vi "SpectrometerSpinCoater_v03_HardwareTrigger.vi"() -> ()   [LabVIEW 2018]
uses:
  <instrlib>/Classes/CCD/Abstract_CCD/Abstract_CCD.lvclass
  TypDef/DeviceQueue_TypeDef.ctl
  TypDef/DeviceQueue_Action.ctl
  TypDef/DataQueue_TypeDef.ctl
  TypDef/DataQueue_Action.ctl
  <vilib>/Utility/error.llb/DialogType.ctl
  <instrlib>/Classes/CCD/Avantes/Avantes.lvclass
  C:/Program Files/National Instruments/LabVIEW 2018/instr.lib/Classes/CCD/Abstract_CCD/Abstract_CCD.lvclass
  <vilib>/Instr/_visa.llb/VISA Configure Serial Port (Instr).vi
panel:
  out "Time.spin":refnum<file>
  out "Meas.spin":refnum<file>
  out "Arduino":bool
  out "NKT":bool
  out "Spectromter":bool
  in  "Abort Button":bool
  in  "Stop Button":bool
  in  "Tab Control":enum32{"Measure", "Settings"}(tab)=enum."Settings"
  out "Action":string
  in  "Preview":bool
  out "XY Graph":T1(graph)
  in  "Frames for Dark/Ref":dbl=1.0
  in  "StartSpin_Button":bool
  out "Overall Time":dbl
  in  "Seconds after Spin Stop":dbl[unit]=0.5
  in  "Program Spin Coater\nSpeed (rpm)          Time (s)":dbl[][](array[numeric])
  in  "Record RefSpec":bool
  in  "Record_Darkspec":bool
  in  "Comments":string="Just for testing"
  in  "File Name":string="Temp"
  in  "Save Path":path=path "C:/Users/Timo/Desktop/SpinCoater/Measurement"
  in  "Seconds to Spin Start":dbl[unit]=1.0
  in  "Calculate Frames":bool=TRUE
  in  "Frames":i32
  out "Frame Rate":dbl[unit]
  in  "Integration Time":dbl[unit]=3e-05
  in  "StartMeasurement_Button":bool
  in  "Speed":dbl
  in  "Milliseconds":dbl
  in  "Debug":bool
  in  "Port Arduino":refnum<visa-resource-name>="COM6"
  out "Error Arduino":bool caption="Error"
  in  "Init_Arduino":bool=TRUE caption="Init"
  out "Caption_Settings_Arduino":string="Arduino"
  out "Caption_Settings_NKT":string="NKT Laser"
  out "Error_Spectromter":bool caption="Error"
  in  "Init_Spectrometer":bool=TRUE caption="Init"
  out "Caption_Settings_Spectrometer":string="Spectromter"
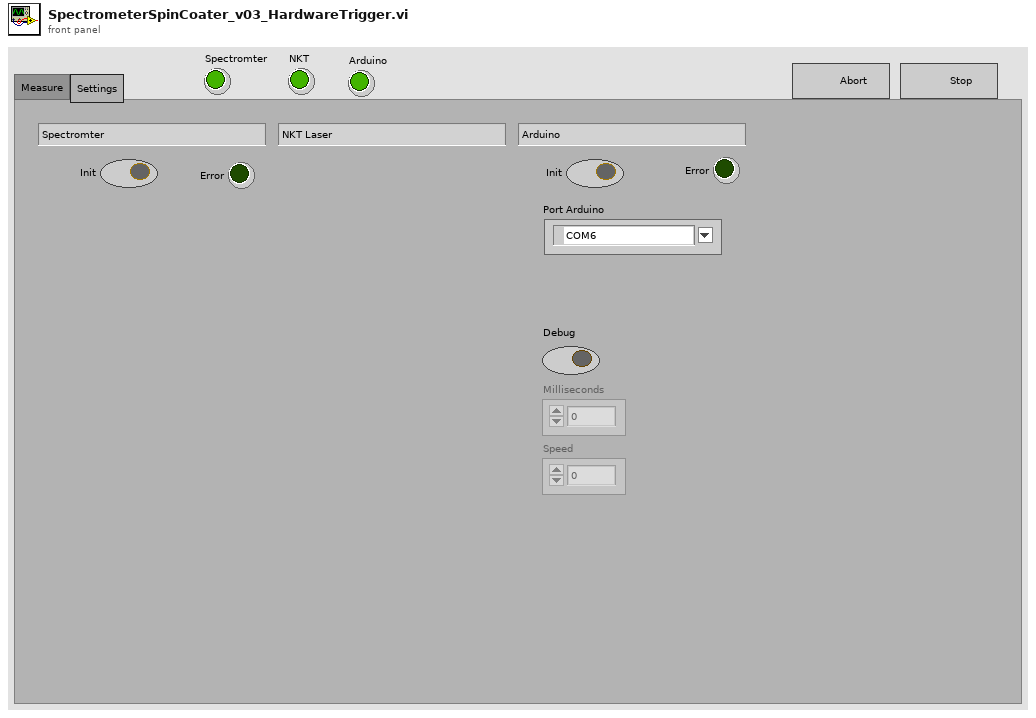
[diagram p1: front panel]
types:
  T1 = cluster{"Wavlength":dbl[unit][], "Image":dbl[]}[]
  T2 = cluster{"Dark":cluster{"Image":dbl[][][], "Frame Size":cluster{"F":i32, "Y":i32, "X":i32}}[], "Ref":cluster{"Image":dbl[][][], "Frame Size":cluster{"F":i32, "Y":i32, "X":i32}}[], "Wavlength":dbl[unit][], "spec":dbl[][]}
  T3 = cluster{"Port Arduino":refnum<visa-resource-name>, "Abstract_CCD.lvclass":refnum<class "Abstract_CCD.lvclass">}
  T4 = typedef "DataQueue_TypeDef.ctl" = cluster{"QueueAction":T5, "Data":cluster{"Image":dbl[][][], "Frame Size":cluster{"F":i32, "Y":i32, "X":i32}}[], "Data_Raw":cluster{"Image":dbl[][][], "Frame Size":cluster{"F":i32, "Y":i32, "X":i32}}[], "Data_Dark":cluster{"Image":dbl[][][], "Frame Size":cluster{"F":i32, "Y":i32, "X":i32}}[], "Data_Ref":cluster{"Image":dbl[][][], "Frame Size":cluster{"F":i32, "Y":i32, "X":i32}}[], "Device Information":string[], "Numeric Control":dbl, "Boolean":bool, "Wavelength":dbl[unit][], "Time":dbl[], "Time Stamp":timestamp, "Numeric Control 2":dbl}
  T5 = typedef "DataQueue_Action.ctl" = enum16{"TimeOut", "Close_Program", "Stop_Measurement", "Measure_InSituSpinCoating", "Save_Data", "Set_Ref", "Set_Dark", "Set_Wavelength", "Spectrometer_Measure", "Transfer_Settings"}
  T6 = typedef "DeviceQueue_TypeDef.ctl" = cluster{"QueueAction":T7, "Numeric 1":dbl, "Numeric 2":dbl, "Boolean 1":bool, "Boolean 2":bool, "Spin Program":dbl[][]}
  T7 = typedef "DeviceQueue_Action.ctl" = enum16{"TimeOut", "Close_Program", "Abort", "Spectrometer_Init", "Spectrometer_Close", "Spectrometer_StartMeasurement", "Spectrometer_StopMeasurement", "Spectrometer_GetData", "Spectrometer_Measure", "Spectrometer_Preview", "Spectrometer_Abort", "Spectrometer_SetIntegrationTime", "Spectrometer_SetFrames", "Spectrometer_SetDarkspec", "Spectrometer_SetReference", "Spectrometer_SetTriggerMode", "Spectrometer_DeviceInformation", "Laser_Init", "Laser_Close", "Arduino_Init", "Arduino_Close", "Arduino_LoadProgram", "Arduino_StartProgram", "Arduino_SetSpeed", "Arduino_SetMillis", "Arduino_StopSpin", "Measure_InSitu", "Measure_Stop"}
  T8 = enum16{"open", "replace", "create", "open or create", "replace or create", "replace or create with confirmation"}
  T9 = cluster{"Image":dbl[][][], "Frame Size":cluster{"F":i32, "Y":i32, "X":i32}}[]
  T10 = cluster{"Image":dbl[][][], "Frame Size":cluster{"F":i32, "Y":i32, "X":i32}}
  T11 = cluster{"Image":dbl[], "Image":dbl[], dbl[], "Numeric Control":dbl, "Numeric Control 2":dbl}
  T12 = typedef "DialogType.ctl" = u16
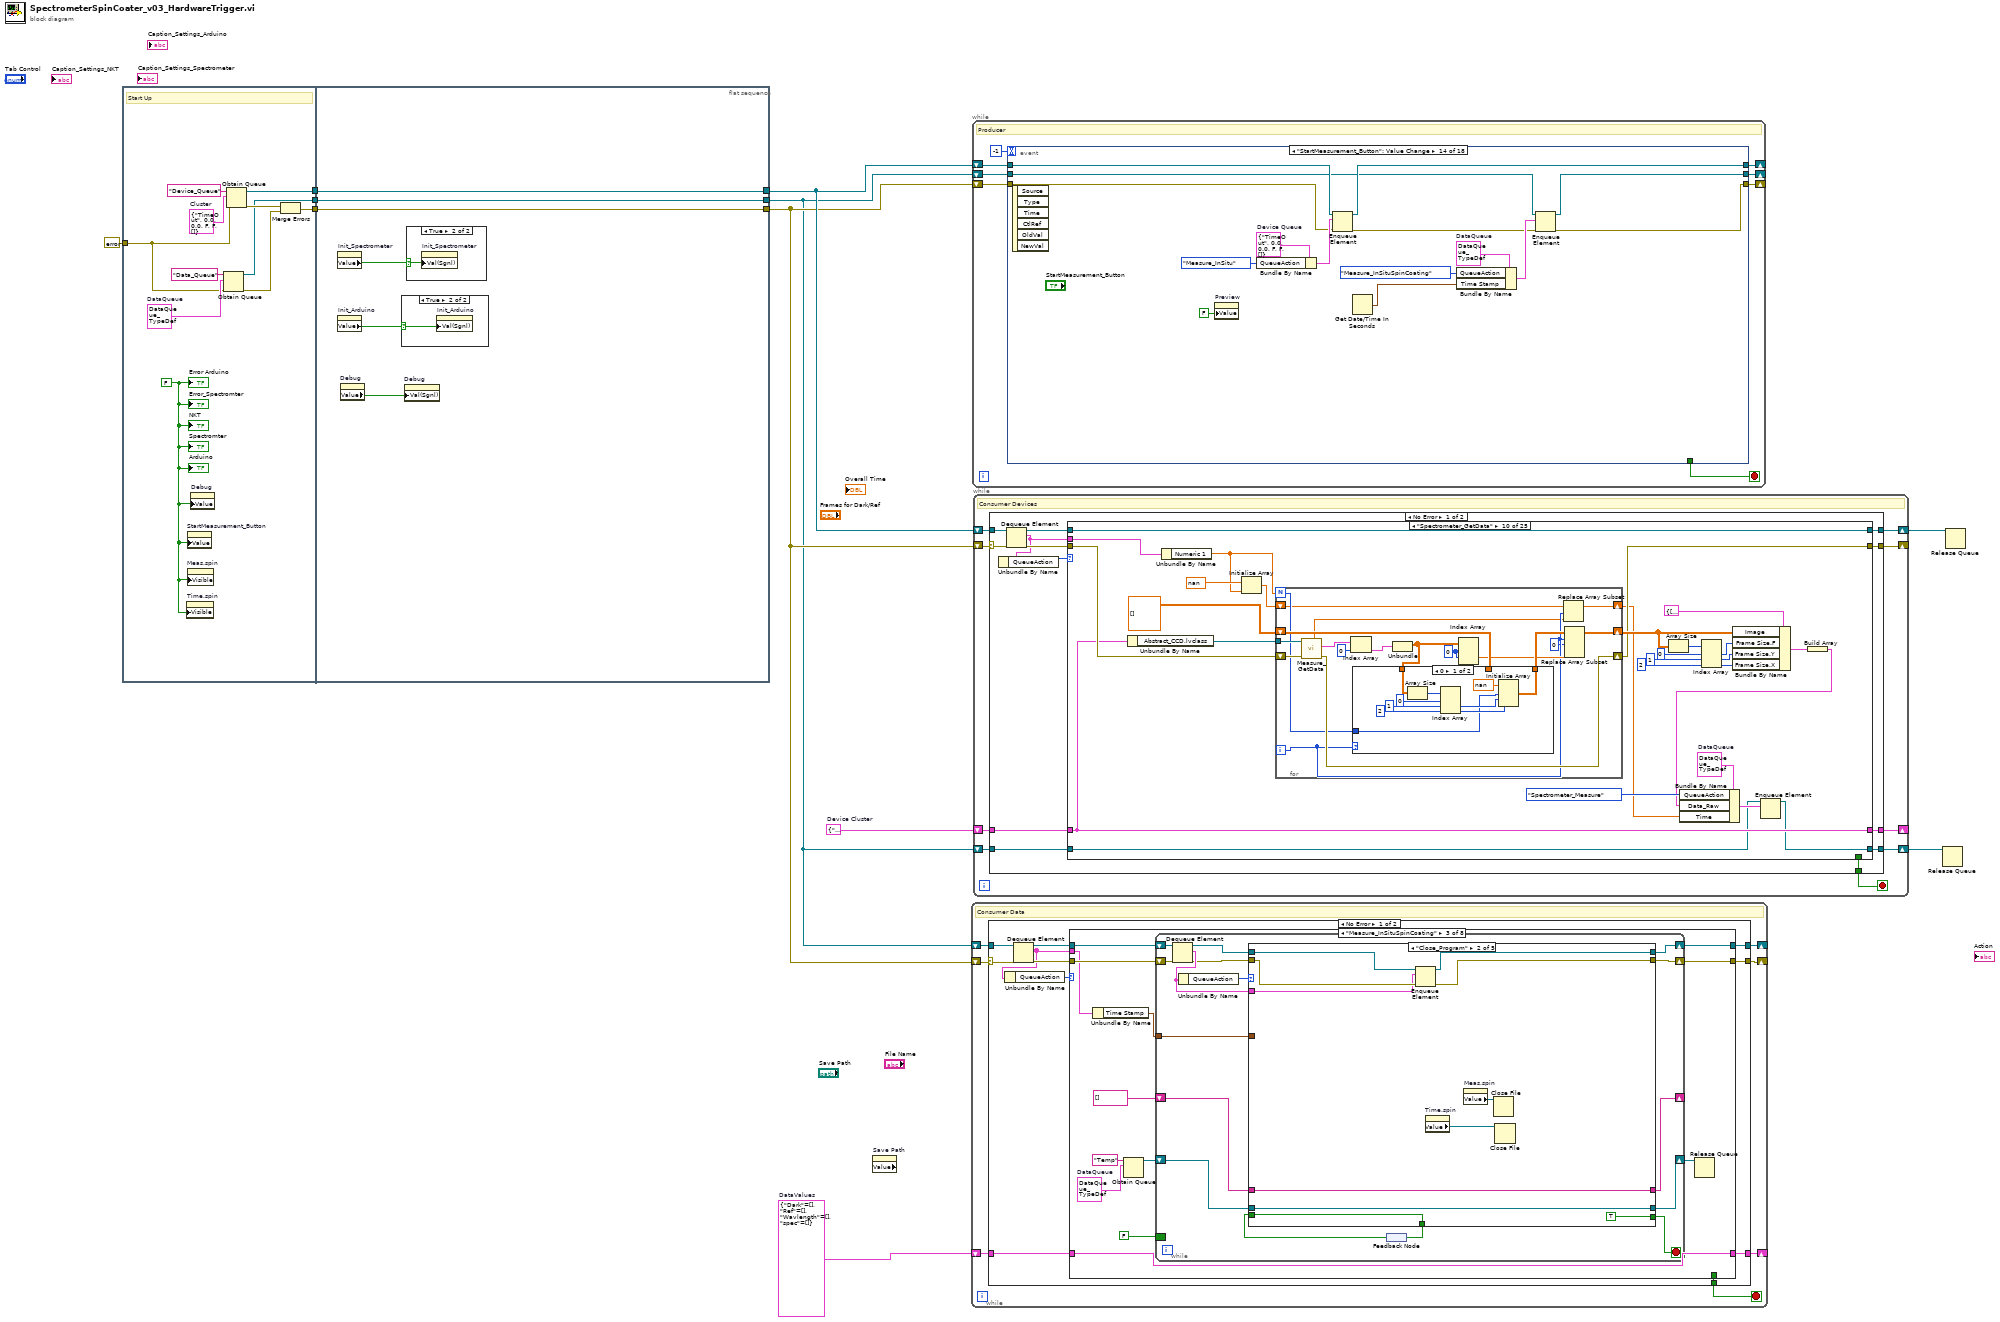
[diagram p0: block diagram]
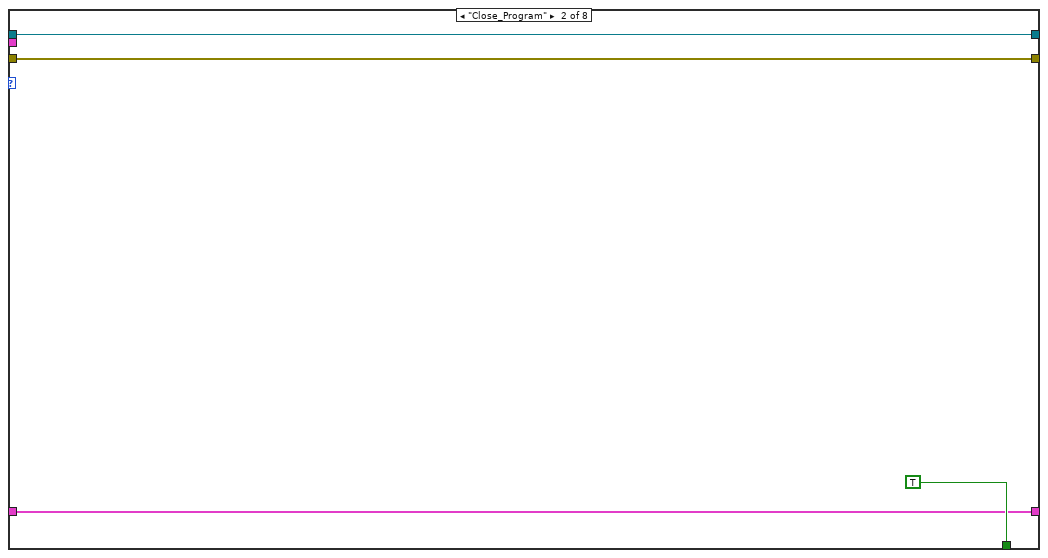
[diagram p5: hidden frame]
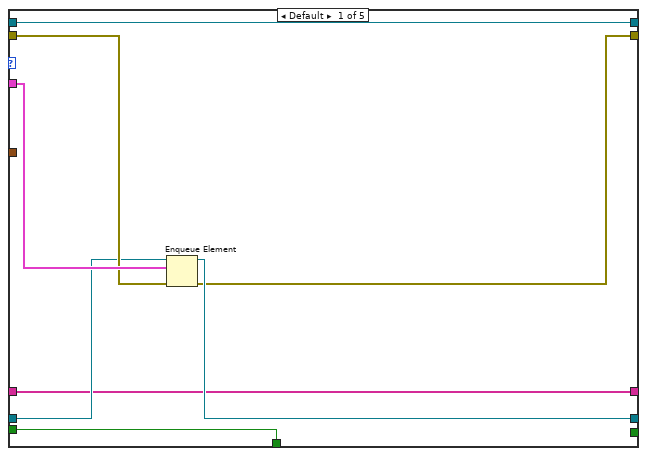
[diagram p6: hidden frame]
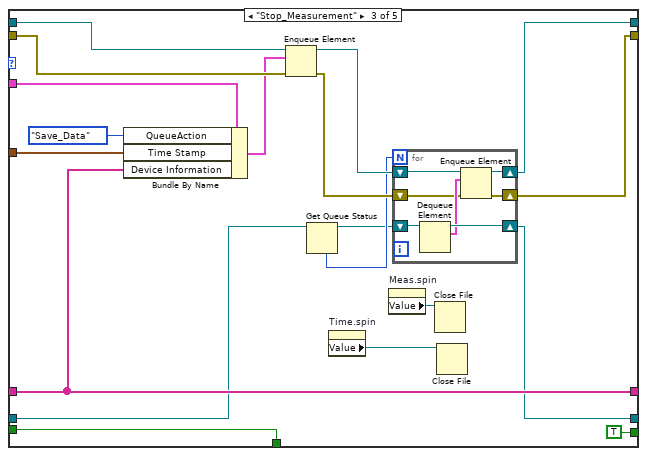
[diagram p7: hidden frame]
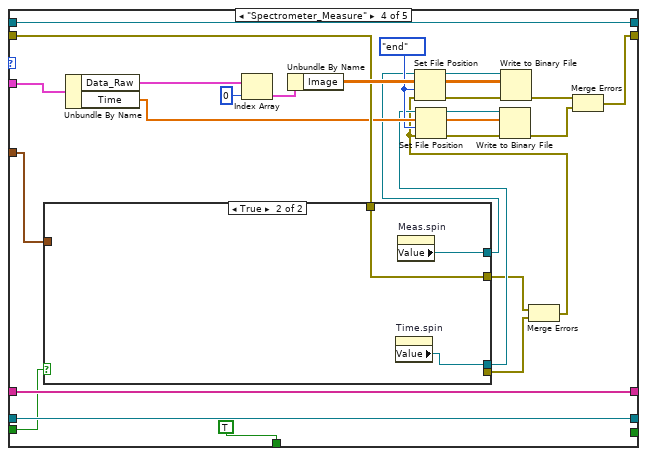
[diagram p8: hidden frame]
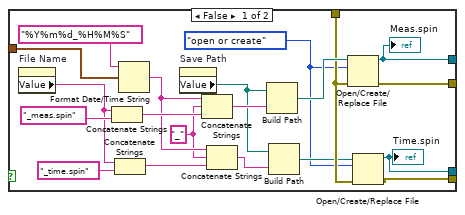
[diagram p9: hidden frame]
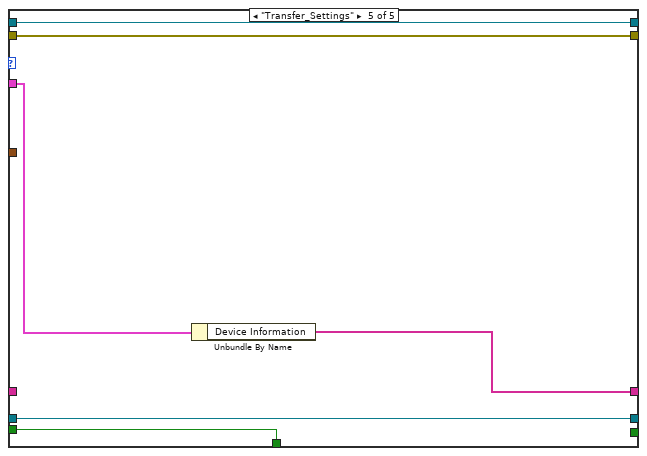
[diagram p10: hidden frame]
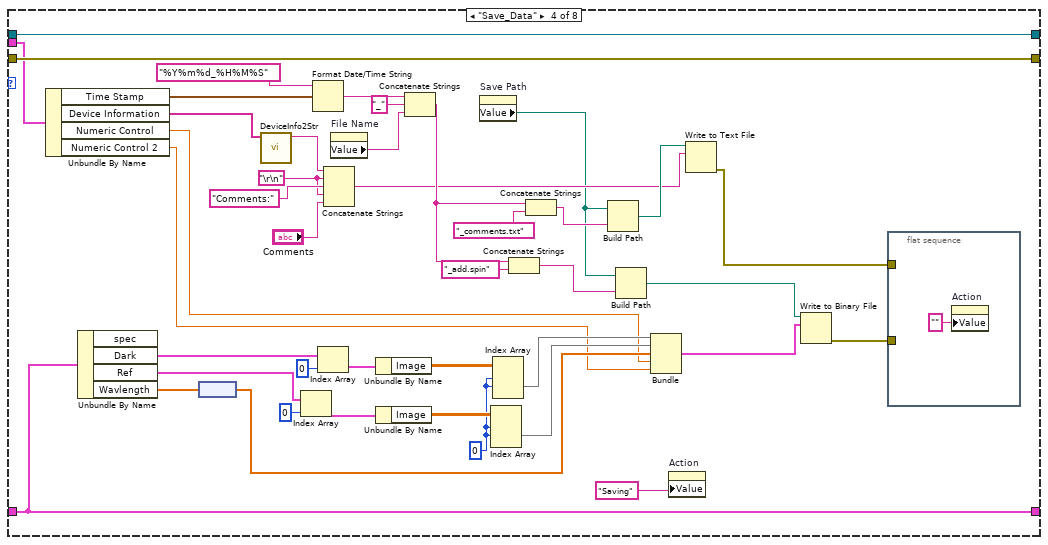
[diagram p11: hidden frame]
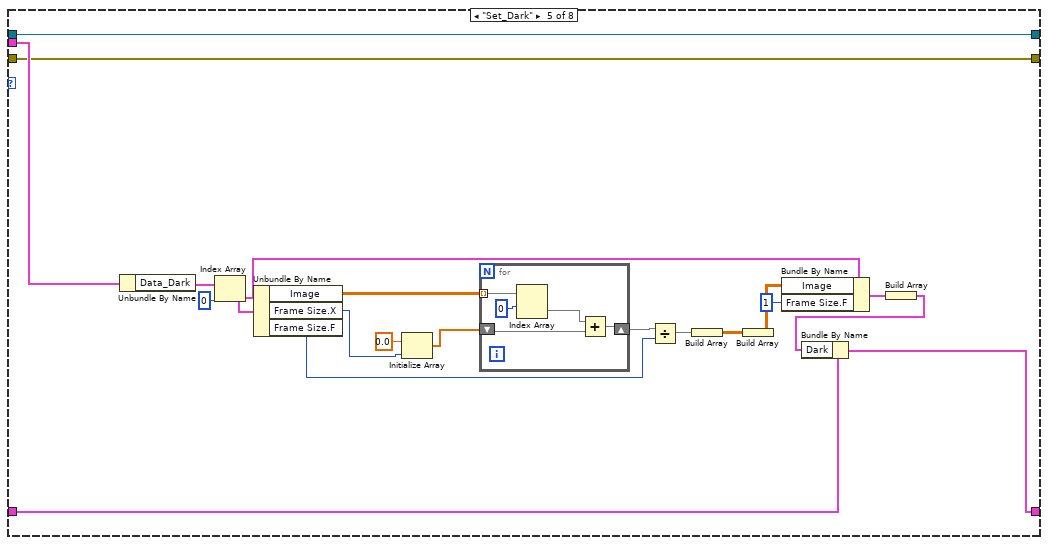
[diagram p12: hidden frame]
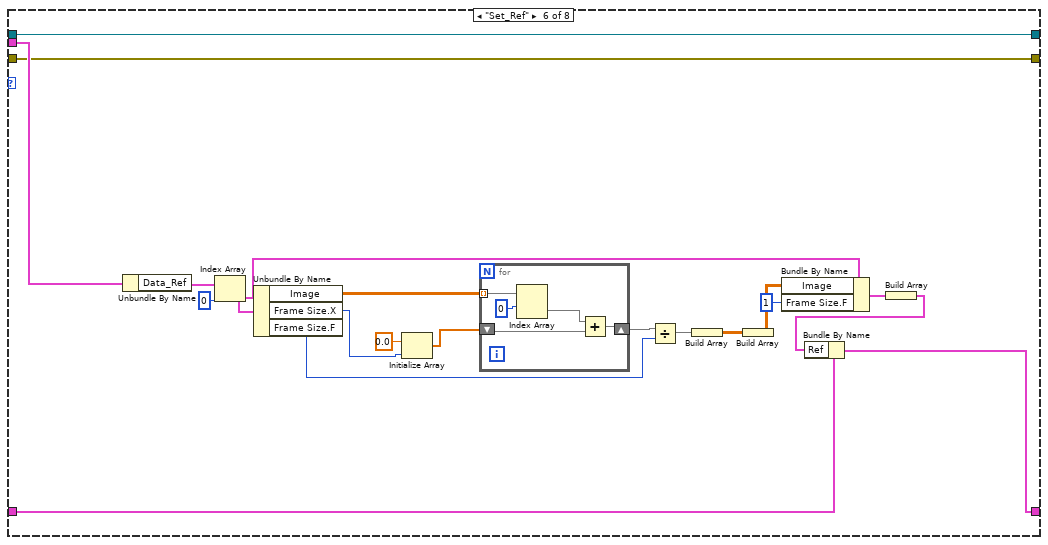
[diagram p13: hidden frame]
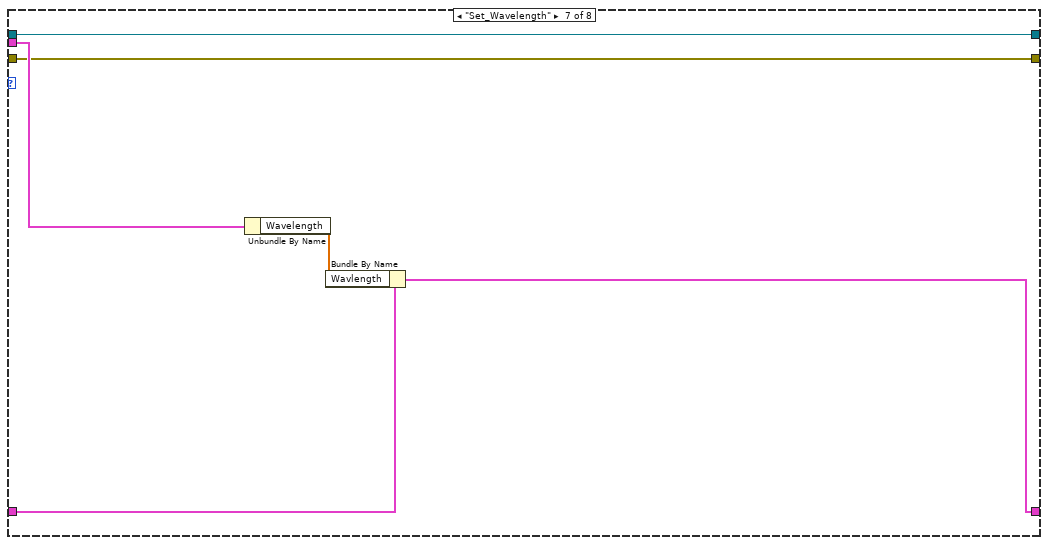
[diagram p14: hidden frame]
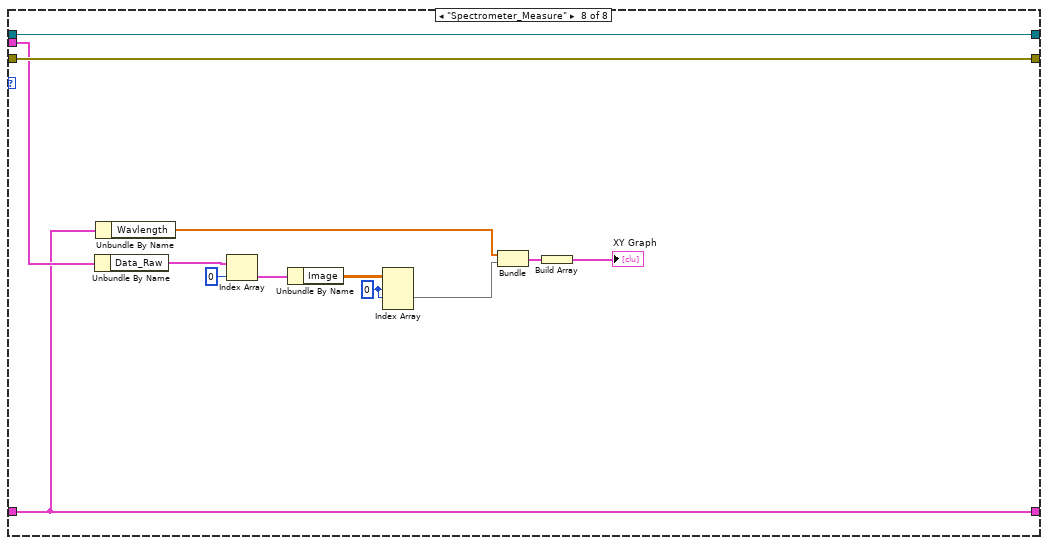
[diagram p15: hidden frame]
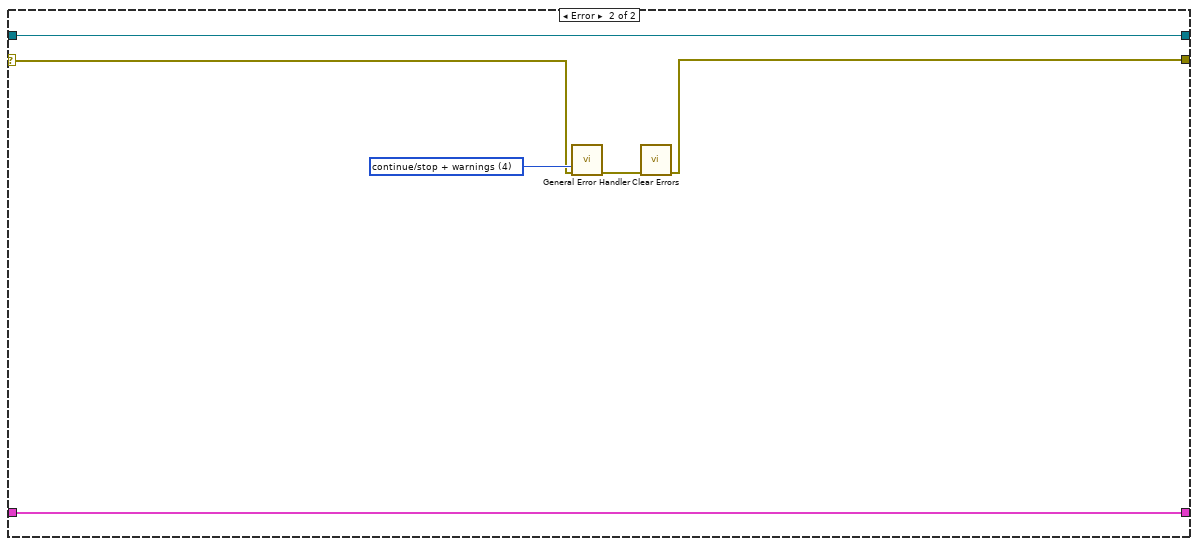
[diagram p16: hidden frame]
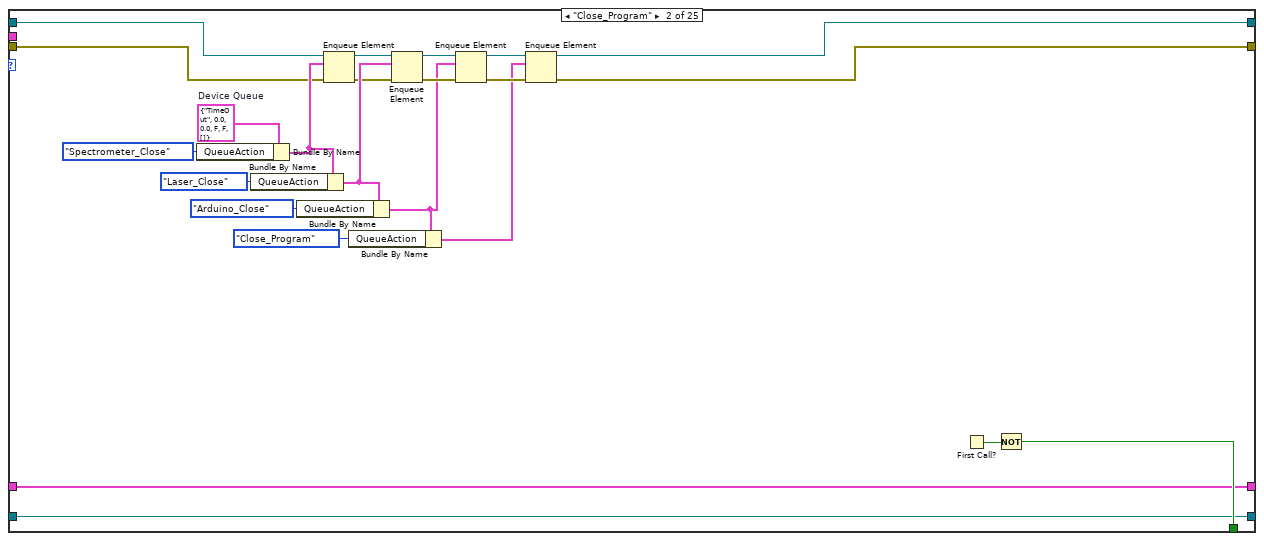
[diagram p18: hidden frame]
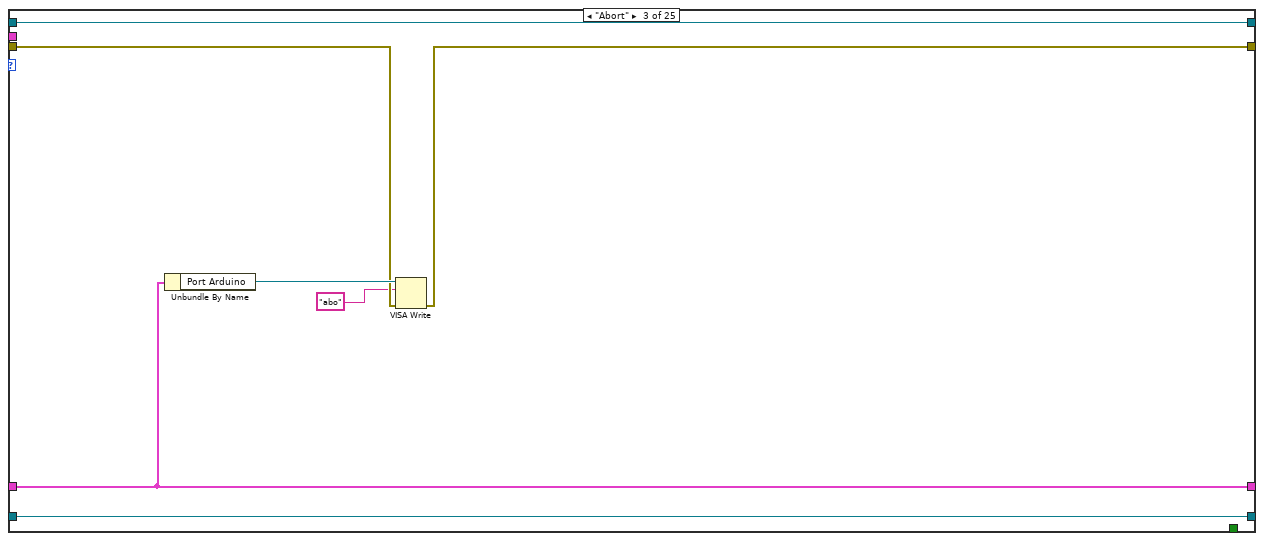
[diagram p19: hidden frame]
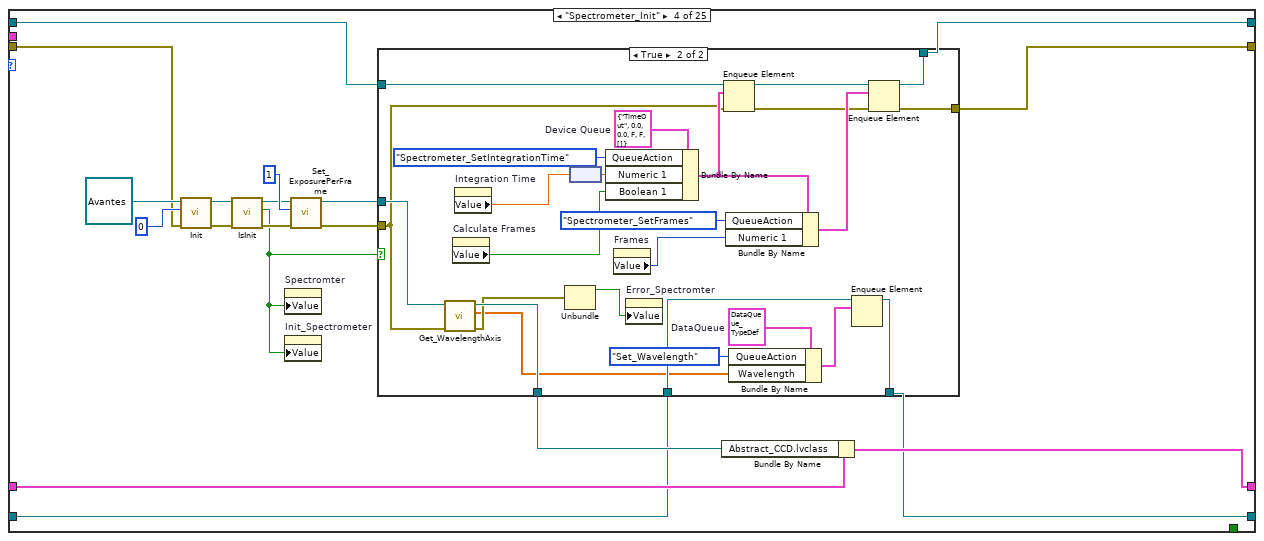
[diagram p20: hidden frame]
diagram:
  w1 = T2 {"Dark"=[], "Ref"=[], "Wavlength"=[], "spec"=[]}  # DataValues
  w6 = T3 {"Port Arduino"="", "Abstract_CCD.lvclass"=refnum}  # Device Cluster
  n1 = flat-sequence {
    tunnel: errorcluster {"status"=FALSE, "code"=0, "source"=""} ("error constant") -> [w17]
    tunnel: [w20] -> w10
    tunnel: [w14] -> w9
    tunnel: [w13] -> w8
    tunnel: w10 -> [w26]
    tunnel: w9 -> [w25]
    tunnel: w8 -> [w24]
    tunnel: [w26] -> w7
    tunnel: [w25] -> w2
    tunnel: [w24] -> w3
    frame #0 {
      w18 = T4 {"QueueAction"=enum."TimeOut", "Data"=[], "Data_Raw"=[], "Data_Dark"=[], "Data_Ref"=[], "Device Information"=[], "Numeric Control"=0.0, "Boolean"=FALSE, "Wavelength"=[], "Time"=[], "Time Stamp"=timestamp(0 s since 1904-01-01), "Numeric Control 2"=0.0}  # DataQueue
      w21 = T6 {"QueueAction"=enum."TimeOut", "Numeric 1"=0.0, "Numeric 2"=0.0, "Boolean 1"=FALSE, "Boolean 2"=FALSE, "Spin Program"=[]}  # Cluster
      w12 = FALSE ("Error Arduino")
      # "Start Up"
      n2 = property on="Time.spin" class="Ref (strict)"("Visible"=w12) -> ()  [unwired: 2 in, 2 out]
      n3 = property on="StartMeasurement_Button" class="Bool (strict)"("Value"=w12) -> ()  [unwired: 2 in, 2 out]
      n4 = property on="Meas.spin" class="Ref (strict)"("Visible"=w12) -> ()  [unwired: 2 in, 2 out]
      n5 = property on="Debug" class="Bool (strict)"("Value"=w12) -> ()  [unwired: 2 in, 2 out]
      n6 = Obtain Queue(name (unnamed)="Data_Queue", element data type=w18, error in (no error)=w17) -> (queue out=w14:refnum<queue>, error out=w15:errorcluster)  [unwired: 2 in, 1 out]
      n7 = Obtain Queue(name (unnamed)="Device_Queue", element data type=w21, error in (no error)=w17) -> (queue out=w20:refnum<queue>, error out=w16:errorcluster)  [unwired: 2 in, 1 out]
      n8 = Merge Errors(w16, w15) -> (w13:errorcluster)
      "Error_Spectromter" <- w12
      "Error Arduino" <- w12
      "Spectromter" <- w12
      "NKT" <- w12
      "Arduino" <- w12
    }
    frame #1 {
      n9 = property on="Init_Spectrometer" class="Bool (strict)"() -> ("Value"=w28:bool)  [unwired: 2 in, 2 out]
      n10 = property on="Init_Arduino" class="Bool (strict)"() -> ("Value"=w27:bool)  [unwired: 2 in, 2 out]
      n11 = property on="Debug" class="Bool (strict)"() -> ("Value"=w23:bool)  [unwired: 2 in, 2 out]
      n12 = case shown="True" w27 {
        selector: w27 -> [_ w29]
        frame False {
        }
        frame True {
          n13 = property on="Init_Arduino" class="Bool (strict)"("Val(Sgnl)"=w29) -> ()  [unwired: 2 in, 2 out]
        }
      }
      n14 = property on="Debug" class="Bool (strict)"("Val(Sgnl)"=w23) -> ()  [unwired: 2 in, 2 out]
      n15 = case shown="True" w28 {
        selector: w28 -> [_ w30]
        frame False {
        }
        frame True {
          n16 = property on="Init_Spectrometer" class="Bool (strict)"("Val(Sgnl)"=w30) -> ()  [unwired: 2 in, 2 out]
        }
      }
    }
  }
  n17 = property on="Save Path" class="Path" props=["Value"]() -> ()  [unwired: 2 in, 3 out]
  n18 = while {
    shift-right: [w31] -> _
    shift-left: w3 -> [w37]
    shift-right: [w32] -> _
    shift-left: w2 -> [w36]
    shift-right: [w33] -> _
    shift-left: w1 -> [w35]
    stop <- w34 stop-if-true
    # "Consumer Data"
    n19 = case shown="No Error" w37 {
      selector: w37 -> [w48 w299]
      tunnel: w36 -> [w47 w300]
      tunnel: w35 -> [w45 w297]
      tunnel: [w44 _] -> w34
      tunnel: [w43 w297] -> w33
      tunnel: [w42 w300] -> w32
      tunnel: [w40 w298] -> w31
      frame No Error {
        n20 = Dequeue Element(queue=w47, error in (no error)=w48) -> (queue out=w41:refnum<queue>, element=w38:T4, error out=w39:errorcluster)  [unwired: 1 in, 1 out]
        n21 = Unbundle By Name(w38) -> ("QueueAction"=w46:T5)
        n22 = case shown="\"Measure_InSituSpinCoating\"" w46 {
          tunnel: w45 -> [w49 w54 w58 w195 w247 w272 w282 w293]
          tunnel: [_ TRUE _ _ _ _ _ _] -> w44
          tunnel: [w49 w54 w58 w195 w243 w268 w281 w293] -> w43
          tunnel: [w51 w53 w68 w226 w244 w269 w278 w296] -> w42
          tunnel: w41 -> [w51 w53 w66 w226 w244 w269 w278 w296]
          tunnel: [w50 w52 w67 w225 w245 w270 w279 w295] -> w40
          tunnel: w39 -> [w50 w52 w65 w225 w245 w270 w279 w295]
          tunnel: w38 -> [_ _ w60 w211 w246 w271 w280 w294]
          frame "TimeOut", Default {
          }
          frame "Close_Program" {
          }
          frame "Measure_InSituSpinCoating" {
            w63 = T4 {"QueueAction"=enum."TimeOut", "Data"=[], "Data_Raw"=[], "Data_Dark"=[], "Data_Ref"=[], "Device Information"=[], "Numeric Control"=0.0, "Boolean"=FALSE, "Wavelength"=[], "Time"=[], "Time Stamp"=timestamp(0 s since 1904-01-01), "Numeric Control 2"=0.0}  # DataQueue
            n23 = Unbundle By Name(w60) -> ("Time Stamp"=w59:timestamp)
            n24 = Obtain Queue(name (unnamed)="Temp", element data type=w63) -> (queue out=w62:refnum<queue>)  [unwired: 3 in, 2 out]
            n25 = while {
              shift-right: [w75] -> w68
              shift-left: w66 -> [w84]
              shift-right: [w76] -> w67
              shift-left: w65 -> [w83]
              shift-right: [w77] -> w61
              shift-left: w62 -> [w78]
              tunnel: w59 -> [w71]
              shift-right: [w72] -> _
              shift-left: string[] [] ("Device Information") -> [w73]
              border: FALSE -> [_]
              stop <- w74 stop-if-true
              n26 = Dequeue Element(queue=w84, error in (no error)=w83) -> (queue out=w79:refnum<queue>, element=w81:T4, error out=w80:errorcluster)  [unwired: 1 in, 1 out]
              n27 = Unbundle By Name(w81) -> ("QueueAction"=w82:T5)
              n28 = feedback #1() -> (w70:bool)
              n29 = case shown="\"Close_Program\"" w82 {
                tunnel: w81 -> [w92 w101 w121 w154 w183]
                tunnel: w80 -> [w91 w102 w118 w144 w180]
                tunnel: w79 -> [w87 w103 w117 w153 w181]
                tunnel: w78 -> [w90 w98 w112 w141 w184]
                tunnel: [w89 w98 w109 w141 w184] -> w77
                tunnel: [w88 w99 w108 w142 w180] -> w76
                tunnel: [w87 w100 w107 w153 w181] -> w75
                tunnel: [_ TRUE TRUE _ _] -> w74
                tunnel: w73 -> [w86 w96 w119 w139 _]
                tunnel: [w86 w96 w119 w139 w182] -> w72
                tunnel: w71 -> [_ _ w120 w155 _]
                tunnel: w70 -> [w85 w95 w106 w137 w179]
                tunnel: [w85 w95 w106 TRUE w179] -> w69
                frame Default {
                  n30 = Enqueue Element(queue=w90, element=w92, error in (no error)=w91) -> (queue out=w89:refnum<queue>, error out=w88:errorcluster)  [unwired: 1 in, 1 out]
                }
                frame "Close_Program" {
                  n31 = Enqueue Element(queue=w103, element=w101, error in (no error)=w102) -> (queue out=w100:refnum<queue>, error out=w99:errorcluster)  [unwired: 1 in, 1 out]
                  n32 = property on="Time.spin" class="Ref (strict)"() -> ("Value"=w93:refnum<file>)  [unwired: 2 in, 2 out]
                  n33 = property on="Meas.spin" class="Ref (strict)"() -> ("Value"=w94:refnum<file>)  [unwired: 2 in, 2 out]
                  n34 = Close File(refnum=w94) -> ()  [unwired: 1 in, 2 out]
                  n35 = Close File(refnum=w93) -> ()  [unwired: 1 in, 2 out]
                }
                frame "Stop_Measurement" {
                  n36 = Bundle By Name(cluster=w121, "QueueAction"=DataQueue_Action."Save_Data", "Time Stamp"=w120, "Device Information"=w119) -> (w116:T4)
                  n37 = Enqueue Element(queue=w117, element=w116, error in (no error)=w118) -> (queue out=w114:refnum<queue>, error out=w113:errorcluster)  [unwired: 1 in, 1 out]
                  n38 = Get Queue Status(queue=w112) -> (queue out=w110:refnum<queue>, # elements in queue=w111:i32)  [unwired: 2 in, 6 out]
                  n39 = property on="Time.spin" class="Ref (strict)"() -> ("Value"=w104:refnum<file>)  [unwired: 2 in, 2 out]
                  n40 = property on="Meas.spin" class="Ref (strict)"() -> ("Value"=w105:refnum<file>)  [unwired: 2 in, 2 out]
                  n41 = for {
                    N: w111 -> [_]
                    shift-right: [w128] -> w109
                    shift-left: w110 -> [w129]
                    shift-right: [w125] -> w107
                    shift-left: w114 -> [w126]
                    shift-right: [w123] -> w108
                    shift-left: w113 -> [w124]
                    n42 = Dequeue Element(queue=w129) -> (queue out=w128:refnum<queue>, element=w127:T4)  [unwired: 2 in, 2 out]
                    n43 = Enqueue Element(queue=w126, element=w127, error in (no error)=w124) -> (queue out=w125:refnum<queue>, error out=w123:errorcluster)  [unwired: 1 in, 1 out]
                  }
                  n44 = Close File(refnum=w105) -> ()  [unwired: 1 in, 2 out]
                  n45 = Close File(refnum=w104) -> ()  [unwired: 1 in, 2 out]
                }
                frame "Spectrometer_Measure" {
                  w140 = enum16{"start", "end", "current"}."end" ("from (0:start)")
                  n46 = case shown="True" w137 {
                    tunnel: w155 -> [w172 _]
                    tunnel: w144 -> [w167 w178]
                    tunnel: [w160 w178] -> w131
                    tunnel: [w159 _] -> w132
                    tunnel: [w158 w177] -> w134
                    tunnel: [w157 w176] -> w133
                    frame False {
                      w161 = T8."open or create" ("operation (0:open)")
                      w156 = "_" ("string")
                      n47 = property on="File Name" class="Str"() -> ("Value"=w170:string)  [unwired: 2 in, 2 out]
                      n48 = Concatenate Strings(w170, "_meas.spin" ("string")) -> (w173:string)
                      n49 = Concatenate Strings(w170, "_time.spin" ("string")) -> (w165:string)
                      n50 = Format Date/Time String(time format string (%c)="%Y%m%d_%H%M%S", seconds (now)=w172) -> (date/time string=w166:string)  [unwired: 1 in]
                      n51 = property on="Save Path" class="Path"() -> ("Value"=w163:path)  [unwired: 2 in, 2 out]
                      n52 = Concatenate Strings(w166, w156, w173) -> (w171:string)
                      n53 = Concatenate Strings(w166, w156, w165) -> (w164:string)
                      n54 = Build Path(base path=w163, name or relative path=w171) -> (appended path=w168:path)
                      n55 = Build Path(base path=w163, name or relative path=w164) -> (appended path=w162:path)
                      n56 = Open/Create/Replace File(file path (use dialog)=w168, error in=w167, operation (0:open)=w161) -> (refnum out=w158:refnum<file>, error out=w160:errorcluster)  [unwired: 3 in, 1 out]
                      "Meas.spin" <- w158
                      n57 = Open/Create/Replace File(file path (use dialog)=w162, error in=w167, operation (0:open)=w161) -> (refnum out=w157:refnum<file>, error out=w159:errorcluster)  [unwired: 3 in, 1 out]
                      "Time.spin" <- w157
                    }
                    frame True {
                      n58 = property on="Time.spin" class="Ref (strict)"() -> ("Value"=w176:refnum<file>)  [unwired: 2 in, 2 out]
                      n59 = property on="Meas.spin" class="Ref (strict)"() -> ("Value"=w177:refnum<file>)  [unwired: 2 in, 2 out]
                    }
                  }
                  n60 = Unbundle By Name(w154) -> ("Data_Raw"=w150:T9, "Time"=w143:dbl[])
                  n61 = Index Array(array=w150, index=0) -> (element=w149:T10)
                  n62 = Unbundle By Name(w149) -> ("Image"=w147:dbl[][][])
                  n63 = Merge Errors(w131, w132) -> (w130:errorcluster)
                  n64 = Set File Position(refnum=w134, from (0:start)=w140, error in=w130) -> (refnum out=w146:refnum<file>, error out=w145:errorcluster)  [unwired: 1 in]
                  n65 = Set File Position(refnum=w133, from (0:start)=w140, error in=w130) -> (refnum out=w152:refnum<file>, error out=w151:errorcluster)  [unwired: 1 in]
                  n66 = Write to Binary File(file (use dialog)=w152, data=w143, error in=w151) -> (error out=w135:errorcluster)  [unwired: 3 in, 2 out]
                  n67 = Write to Binary File(file (use dialog)=w146, data=w147, error in=w145) -> (error out=w136:errorcluster)  [unwired: 3 in, 2 out]
                  n68 = Merge Errors(w136, w135) -> (w142:errorcluster)
                }
                frame "Transfer_Settings" {
                  n69 = Unbundle By Name(w183) -> ("Device Information"=w182:string[])
                }
              }
              n70 = feedback-in #1(w69) -> ()
            }
            n71 = Release Queue(queue=w61) -> ()  [unwired: 2 in, 3 out]
          }
          frame "Save_Data" {
            w197 = "\r\n"
            w215 = 0 ("index (page)")
            n72 = Unbundle By Name(w211) -> ("Time Stamp"=w209:timestamp, "Device Information"=w200:string[], "Numeric Control"=w194:dbl, "Numeric Control 2"=w193:dbl)
            n73 = Unbundle By Name(w195) -> ("Dark"=w222:T9, "Ref"=w220:T9, "Wavlength"=w224:dbl[unit][])  [unwired: 1 out]
            n74 = node(w224) -> (w212:dbl[])
            n75 = call "DeviceInfo2Str.vi"("Device Information"=w200) -> ("String"=w199:string)  [unwired: 10 in]
            n76 = Index Array(array=w220, index=0) -> (element=w218:T10)
            n77 = Format Date/Time String(time format string (%c)="%Y%m%d_%H%M%S", seconds (now)=w209) -> (date/time string=w208:string)  [unwired: 1 in]
            n78 = Index Array(array=w222, index=0) -> (element=w219:T10)
            n79 = Concatenate Strings(w199, w197, "Comments:" ("string"), w197, "Comments") -> (w192:string)
            n80 = property on="File Name" class="Str"() -> ("Value"=w190:string)  [unwired: 2 in, 2 out]
            n81 = Unbundle By Name(w219) -> ("Image"=w217:dbl[][][])
            n82 = Unbundle By Name(w218) -> ("Image"=w216:dbl[][][])
            n83 = Concatenate Strings(w208, "_" ("string"), w190) -> (w206:string)
            n84 = property on="Save Path" class="Path"() -> ("Value"=w189:path)  [unwired: 2 in, 2 out]
            n85 = Index Array(array=w216, index (dim 0)=w215, index (dim 1)=w215) -> (element=w213:dbl[])  [unwired: 1 in]
            n86 = Index Array(array=w217, index (dim 0)=w215, index (dim 1)=w215) -> (element=w214:dbl[])  [unwired: 1 in]
            n87 = Concatenate Strings(w206, "_add.spin" ("string")) -> (w204:string)
            n88 = Concatenate Strings(w206, "_comments.txt" ("string")) -> (w203:string)
            n89 = Build Path(base path=w189, name or relative path=w203) -> (appended path=w202:path)
            n90 = Build Path(base path=w189, name or relative path=w204) -> (appended path=w188:path)
            n91 = Bundle("Image"=w214, "Image"=w213, w212, "Numeric Control"=w194, "Numeric Control 2"=w193) -> (w187:T11)  [unwired: 1 in]
            n92 = property on="Action" class="Str"("Value"="Saving" ("Action")) -> ()  [unwired: 2 in, 2 out]
            n93 = Write to Text File(file (use dialog)=w202, text=w192) -> (error out=w186:errorcluster)  [unwired: 2 in, 2 out]
            n94 = Write to Binary File(file (use dialog)=w188, data=w187) -> (error out=w185:errorcluster)  [unwired: 4 in, 2 out]
            n95 = flat-sequence {
              tunnel: w186 -> [_]
              tunnel: w185 -> [_]
              frame #0 {
                n96 = property on="Action" class="Str"("Value"="" ("Action")) -> ()  [unwired: 2 in, 2 out]
              }
            }
          }
          frame "Set_Dark" {
            n97 = Unbundle By Name(w246) -> ("Data_Dark"=w233:T9)
            n98 = Index Array(array=w233, index=0) -> (element=w232:T10)
            n99 = Unbundle By Name(w232) -> ("Image"=w241:dbl[][][], "Frame Size.X"=w239:i32, "Frame Size.F"=w236:i32)
            n100 = Initialize Array(0.0 ("element"), w239) -> (w238:dbl[])
            n101 = for {
              tunnel: w241 -> [w252] mode=indexing
              shift-right: [w248] -> w237
              shift-left: w238 -> [w249]
              n102 = Index Array(array=w252, index (row)=0) -> (element=w250:dbl[])  [unwired: 1 in]
              n103 = Add(x=w250, y=w249) -> (x+y=w248:dbl[])
            }
            n104 = Divide(x=w237, y=w236) -> (x/y=w235:dbl[])
            n105 = Build Array(w235) -> (w234:dbl[][])
            n106 = Build Array(w234) -> (w231:dbl[][][])
            n107 = Bundle By Name(cluster=w232, "Image"=w231, "Frame Size.F"=1) -> (w229:T10)
            n108 = Build Array(w229) -> (w228:T9)
            n109 = Bundle By Name(cluster=w247, "Dark"=w228) -> (w243:T2)
          }
          frame "Set_Ref" {
            n110 = Unbundle By Name(w271) -> ("Data_Ref"=w258:T9)
            n111 = Index Array(array=w258, index=0) -> (element=w257:T10)
            n112 = Unbundle By Name(w257) -> ("Image"=w266:dbl[][][], "Frame Size.X"=w264:i32, "Frame Size.F"=w261:i32)
            n113 = Initialize Array(0.0 ("element"), w264) -> (w263:dbl[])
            n114 = for {
              tunnel: w266 -> [w277] mode=indexing
              shift-right: [w273] -> w262
              shift-left: w263 -> [w274]
              n115 = Index Array(array=w277, index (row)=0) -> (element=w275:dbl[])  [unwired: 1 in]
              n116 = Add(x=w275, y=w274) -> (x+y=w273:dbl[])
            }
            n117 = Divide(x=w262, y=w261) -> (x/y=w260:dbl[])
            n118 = Build Array(w260) -> (w259:dbl[][])
            n119 = Build Array(w259) -> (w256:dbl[][][])
            n120 = Bundle By Name(cluster=w257, "Image"=w256, "Frame Size.F"=1) -> (w254:T10)
            n121 = Build Array(w254) -> (w253:T9)
            n122 = Bundle By Name(cluster=w272, "Ref"=w253) -> (w268:T2)
          }
          frame "Set_Wavelength" {
            n123 = Unbundle By Name(w280) -> ("Wavelength"=w283:dbl[unit][])
            n124 = Bundle By Name(cluster=w282, "Wavlength"=w283) -> (w281:T2)
          }
          frame "Spectrometer_Measure" {
            w288 = 0 ("index (page)")
            n125 = Unbundle By Name(w294) -> ("Data_Raw"=w292:T9)
            n126 = Unbundle By Name(w293) -> ("Wavlength"=w287:dbl[unit][])
            n127 = Index Array(array=w292, index=0) -> (element=w290:T10)
            n128 = Unbundle By Name(w290) -> ("Image"=w289:dbl[][][])
            n129 = Index Array(array=w289, index (dim 0)=w288, index (dim 1)=w288) -> (element=w286:dbl[])  [unwired: 1 in]
            n130 = Bundle("Wavlength"=w287, "Image"=w286) -> (w285:cluster{"Wavlength":dbl[unit][], "Image":dbl[]})  [unwired: 1 in]
            n131 = Build Array(w285) -> (→"XY Graph":T1)
          }
        }
      }
      frame Error {
        w302 = T12 4 items=["no dialog", "OK message", "continue or stop message", "OK message + warnings", "continue/stop + warnings"] ("type of dialog (OK msg:1)")
        n132 = call <vilib>:"General Error Handler.vi"("type of dialog (OK msg:1)"=w302, "error in (no error)"=w299) -> ("error out"=w301:errorcluster)  [unwired: 9 in, 4 out]
        n133 = call <vilib>:"Clear Errors.vi"("error in (no error)"=w301) -> ("error out"=w298:errorcluster)  [unwired: 5 in, 1 out]
      }
    }
  }
  n134 = while {
    shift-right: [w305] -> _
    shift-left: w7 -> [w303]
    shift-right: [w308] -> _
    shift-left: w2 -> [w309]
    shift-right: [w306] -> _
    shift-left: w3 -> [w307]
    stop <- w304 stop-if-true
    # "Producer"
    n135 = event shown="[13] \"StartMeasurement_Button\": Value Change" {
      selector: _ -> [_ _ _ _ _ _ _ _ _ _ _ _ _ _ _ _ _ _]
      dyn-events: _ -> [_ _ _ _ _ _ _ _ _ _ _ _ _ _ _ _ _ _]
      timeout: -1 -> [_ _ _ _ _ _ _ _ _ _ _ _ _ _ _ _ _ _]
      tunnel: w309 -> [w312 w327 w331 w343 w356 w371 w383 w394 w397 w404 w423 w430 w439 w447 w462 w472 w481 w489]
      tunnel: [w312 w324 w331 w343 w356 w371 w383 w394 w397 w404 w423 w430 w439 w446 w462 w472 w481 w489] -> w308
      tunnel: w307 -> [w311 w326 w333 w341 w353 w370 w381 w389 w396 w401 w421 w429 w437 w453 w459 w471 w480 w488]
      tunnel: [w311 w320 w330 w337 w352 w368 w379 w388 w396 w399 w420 w427 w436 w445 w460 w468 w477 w488] -> w306
      tunnel: w303 -> [w313 w328 w334 w342 w355 w372 w382 w391 w398 w402 w424 w431 w440 w455 w463 w473 w482 w490]
      tunnel: [w313 w325 w332 w338 w354 w369 w380 w390 w398 w403 w422 w428 w438 w454 w461 w469 w478 w490] -> w305
      tunnel: [_ TRUE _ _ _ _ _ _ _ _ _ _ _ _ _ _ _ _] -> w304
      event Timeout {
        n136 = event-data() -> ()  [unwired: 1 in, 3 out]
      }
      event "Stop Button": Value Change {
        w316 = T4 {"QueueAction"=enum."TimeOut", "Data"=[], "Data_Raw"=[], "Data_Dark"=[], "Data_Ref"=[], "Device Information"=[], "Numeric Control"=0.0, "Boolean"=FALSE, "Wavelength"=[], "Time"=[], "Time Stamp"=timestamp(0 s since 1904-01-01), "Numeric Control 2"=0.0}  # DataQueue
        w319 = T6 {"QueueAction"=enum."TimeOut", "Numeric 1"=0.0, "Numeric 2"=0.0, "Boolean 1"=FALSE, "Boolean 2"=FALSE, "Spin Program"=[]}  # Device Queue
        n137 = event-data() -> ()  [unwired: 1 in, 6 out]
        n138 = Bundle By Name(cluster=w319, "QueueAction"=DeviceQueue_Action."Close_Program") -> (w317:T6)
        n139 = Enqueue Element(queue=w328, element=w317, error in (no error)=w326) -> (queue out=w325:refnum<queue>, error out=w321:errorcluster)  [unwired: 1 in, 1 out]
        n140 = Bundle By Name(cluster=w316, "QueueAction"=DataQueue_Action."Close_Program") -> (w314:T4)
        n141 = Enqueue Element(queue=w327, element=w314, error in (no error)=w326) -> (queue out=w324:refnum<queue>, error out=w322:errorcluster)  [unwired: 1 in, 1 out]
        n142 = Merge Errors(w322, w321) -> (w320:errorcluster)
      }
      event "Abort Button": Value Change {
        w336 = T6 {"QueueAction"=enum."TimeOut", "Numeric 1"=0.0, "Numeric 2"=0.0, "Boolean 1"=FALSE, "Boolean 2"=FALSE, "Spin Program"=[]}  # Device Queue
        # "At the moment just spin coater in non in-situ measurements can be stopped"
        n143 = event-data() -> ()  [unwired: 1 in, 6 out]
        n144 = Bundle By Name(cluster=w336, "QueueAction"=DeviceQueue_Action."Abort") -> (w335:T6)
        n145 = Enqueue Element(queue=w334, element=w335, error in (no error)=w333) -> (queue out=w332:refnum<queue>, error out=w330:errorcluster)  [unwired: 1 in, 1 out]
      }
      event "Init_Spectrometer": Value Change {
        n146 = event-data() -> ()  [unwired: 1 in, 6 out]
        n147 = case shown="False" "Init_Spectrometer" {
          tunnel: [w344 w347] -> w339
          frame True {
            n148 = Bundle By Name(cluster=T6 {"QueueAction"=enum."TimeOut", "Numeric 1"=0.0, "Numeric 2"=0.0, "Boolean 1"=FALSE, "Boolean 2"=FALSE, "Spin Program"=[]} ("element"), "QueueAction"=DeviceQueue_Action."Spectrometer_Init") -> (w344:T6)
          }
          frame False {
            n149 = Bundle By Name(cluster=T6 {"QueueAction"=enum."TimeOut", "Numeric 1"=0.0, "Numeric 2"=0.0, "Boolean 1"=FALSE, "Boolean 2"=FALSE, "Spin Program"=[]} ("element"), "QueueAction"=DeviceQueue_Action."Spectrometer_Close") -> (w347:T6)
          }
        }
        n150 = Enqueue Element(queue=w342, element=w339, error in (no error)=w341) -> (queue out=w338:refnum<queue>, error out=w337:errorcluster)  [unwired: 1 in, 1 out]
      }
      event "Init_Arduino": Value Change {
        n151 = event-data() -> ("NewVal"=w351:bool)  [unwired: 1 in, 5 out]
        n152 = case shown="True" w351 {
          tunnel: [w357 w360] -> w350
          frame False {
            w359 = T6 {"QueueAction"=enum."TimeOut", "Numeric 1"=0.0, "Numeric 2"=0.0, "Boolean 1"=FALSE, "Boolean 2"=FALSE, "Spin Program"=[]}  # Device Queue
            n153 = Bundle By Name(cluster=w359, "QueueAction"=DeviceQueue_Action."Arduino_Close") -> (w357:T6)
          }
          frame True {
            w362 = T6 {"QueueAction"=enum."TimeOut", "Numeric 1"=0.0, "Numeric 2"=0.0, "Boolean 1"=FALSE, "Boolean 2"=FALSE, "Spin Program"=[]}  # Device Queue
            n154 = Bundle By Name(cluster=w362, "QueueAction"=DeviceQueue_Action."Arduino_Init") -> (w360:T6)
          }
        }
        n155 = Enqueue Element(queue=w355, element=w350, error in (no error)=w353) -> (queue out=w354:refnum<queue>, error out=w352:errorcluster)  [unwired: 1 in, 1 out]
      }
      event "Program Spin Coater\nSpeed (rpm)          Time (s)": Value Change {
        w374 = T6 {"QueueAction"=enum."TimeOut", "Numeric 1"=0.0, "Numeric 2"=0.0, "Boolean 1"=FALSE, "Boolean 2"=FALSE, "Spin Program"=[]}  # Device Queue
        n156 = event-data() -> ("NewVal"=w366:dbl[][])  [unwired: 1 in, 5 out]
        n157 = property on="Seconds to Spin Start" class="DigNum (strict)"() -> ("Value"=w364:dbl[unit])  [unwired: 2 in, 2 out]
        n158 = node(w364) -> (w363:dbl)
        n159 = Bundle By Name(cluster=w374, "QueueAction"=DeviceQueue_Action."Arduino_LoadProgram", "Spin Program"=w366, "Numeric 1"=w363) -> (w373:T6)
        n160 = Enqueue Element(queue=w372, element=w373, error in (no error)=w370) -> (queue out=w369:refnum<queue>, error out=w368:errorcluster)  [unwired: 1 in, 1 out]
        n161 = property on="Integration Time" class="DigNum (strict)"() -> ("Value"=w365:dbl[unit])  [unwired: 2 in, 2 out]
        n162 = property on="Integration Time" class="DigNum (strict)"("Val(Sgnl)"=w365) -> ()  [unwired: 2 in, 2 out]
      }
      event "Integration Time": Value Change {
        w385 = T6 {"QueueAction"=enum."TimeOut", "Numeric 1"=0.0, "Numeric 2"=0.0, "Boolean 1"=FALSE, "Boolean 2"=FALSE, "Spin Program"=[]}  # Device Queue
        n163 = event-data() -> ("NewVal"=w377:dbl[unit])  [unwired: 1 in, 5 out]
        n164 = node(w377) -> (w376:dbl)
        n165 = property on="Calculate Frames" class="Bool (strict)"() -> ("Value"=w375:bool)  [unwired: 2 in, 2 out]
        n166 = Bundle By Name(cluster=w385, "QueueAction"=DeviceQueue_Action."Spectrometer_SetIntegrationTime", "Numeric 1"=w376, "Boolean 1"=w375) -> (w384:T6)
        n167 = Enqueue Element(queue=w382, element=w384, error in (no error)=w381) -> (queue out=w380:refnum<queue>, error out=w379:errorcluster)  [unwired: 1 in, 1 out]
      }
      event "Frames": Value Change {
        w393 = T6 {"QueueAction"=enum."TimeOut", "Numeric 1"=0.0, "Numeric 2"=0.0, "Boolean 1"=FALSE, "Boolean 2"=FALSE, "Spin Program"=[]}  # Device Queue
        n168 = event-data() -> ()  [unwired: 1 in, 6 out]
        n169 = Bundle By Name(cluster=w393, "QueueAction"=DeviceQueue_Action."Spectrometer_SetFrames", "Numeric 1"="Frames") -> (w392:T6)
        n170 = Enqueue Element(queue=w391, element=w392, error in (no error)=w389) -> (queue out=w390:refnum<queue>, error out=w388:errorcluster)  [unwired: 1 in, 1 out]
      }
      event "Seconds to Spin Start", "Seconds after Spin Stop": Value Change {
        n171 = event-data() -> ()  [unwired: 1 in, 6 out]
        n172 = property on="Program Spin Coater\nSpeed (rpm)          Time (s)" class="Arr (strict)"() -> ("Value"=w395:dbl[][])  [unwired: 2 in, 2 out]
        n173 = property on="Program Spin Coater\nSpeed (rpm)          Time (s)" class="Arr (strict)"("Val(Sgnl)"=w395) -> ()  [unwired: 2 in, 2 out]
      }
      event "Calculate Frames": Value Change {
        n174 = event-data() -> ("NewVal"=w405:bool)  [unwired: 1 in, 5 out]
        n175 = case shown="False" w405 {
          tunnel: [0 2] -> w400
          tunnel: w402 -> [w407 w416]
          tunnel: [w407 w414] -> w403
          tunnel: w401 -> [w406 w413]
          tunnel: [w406 w409] -> w399
          frame False {
          }
          frame True {
            w415 = T6 {"QueueAction"=enum."TimeOut", "Numeric 1"=0.0, "Numeric 2"=0.0, "Boolean 1"=FALSE, "Boolean 2"=FALSE, "Spin Program"=[]}  # Device Queue
            n176 = property on="Integration Time" class="DigNum (strict)"() -> ("Value"=w411:dbl[unit])  [unwired: 2 in, 2 out]
            n177 = node(w411) -> (w410:dbl)
            n178 = Bundle By Name(cluster=w415, "QueueAction"=DeviceQueue_Action."Spectrometer_SetIntegrationTime", "Numeric 1"=w410) -> (w417:T6)
            n179 = Enqueue Element(queue=w416, element=w417, error in (no error)=w413) -> (queue out=w414:refnum<queue>, error out=w409:errorcluster)  [unwired: 1 in, 1 out]
          }
        }
        n180 = property on="Frames" class="DigNum (strict)"("DisabledEnum"=w400) -> ()  [unwired: 2 in, 2 out]
      }
      event "Record RefSpec": Value Change {
        w426 = T6 {"QueueAction"=enum."TimeOut", "Numeric 1"=0.0, "Numeric 2"=0.0, "Boolean 1"=FALSE, "Boolean 2"=FALSE, "Spin Program"=[]}  # Device Queue
        n181 = event-data() -> ()  [unwired: 1 in, 6 out]
        n182 = Bundle By Name(cluster=w426, "QueueAction"=DeviceQueue_Action."Spectrometer_SetReference") -> (w425:T6)
        n183 = Enqueue Element(queue=w424, element=w425, error in (no error)=w421) -> (queue out=w422:refnum<queue>, error out=w420:errorcluster)  [unwired: 1 in, 1 out]
      }
      event "Preview": Value Change {
        w434 = T6 {"QueueAction"=enum."TimeOut", "Numeric 1"=0.0, "Numeric 2"=0.0, "Boolean 1"=FALSE, "Boolean 2"=FALSE, "Spin Program"=[]}  # Device Queue
        n184 = event-data() -> ()  [unwired: 1 in, 6 out]
        n185 = Bundle By Name(cluster=w434, "QueueAction"=DeviceQueue_Action."Spectrometer_Preview") -> (w433:T6)
        n186 = Enqueue Element(queue=w431, element=w433, error in (no error)=w429) -> (queue out=w428:refnum<queue>, error out=w427:errorcluster)  [unwired: 1 in, 1 out]
      }
      event "Record_Darkspec": Value Change {
        w442 = T6 {"QueueAction"=enum."TimeOut", "Numeric 1"=0.0, "Numeric 2"=0.0, "Boolean 1"=FALSE, "Boolean 2"=FALSE, "Spin Program"=[]}  # Device Queue
        n187 = event-data() -> ()  [unwired: 1 in, 6 out]
        n188 = Bundle By Name(cluster=w442, "QueueAction"=DeviceQueue_Action."Spectrometer_SetDarkspec") -> (w441:T6)
        n189 = Enqueue Element(queue=w440, element=w441, error in (no error)=w437) -> (queue out=w438:refnum<queue>, error out=w436:errorcluster)  [unwired: 1 in, 1 out]
      }
      event "StartMeasurement_Button": Value Change {
        w449 = T4 {"QueueAction"=enum."TimeOut", "Data"=[], "Data_Raw"=[], "Data_Dark"=[], "Data_Ref"=[], "Device Information"=[], "Numeric Control"=0.0, "Boolean"=FALSE, "Wavelength"=[], "Time"=[], "Time Stamp"=timestamp(0 s since 1904-01-01), "Numeric Control 2"=0.0}  # DataQueue
        w457 = T6 {"QueueAction"=enum."TimeOut", "Numeric 1"=0.0, "Numeric 2"=0.0, "Boolean 1"=FALSE, "Boolean 2"=FALSE, "Spin Program"=[]}  # Device Queue
        n190 = event-data() -> ()  [unwired: 1 in, 6 out]
        n191 = property on="Preview" class="Bool (strict)"("Value"=FALSE ("Preview")) -> ()  [unwired: 2 in, 2 out]
        n192 = Bundle By Name(cluster=w457, "QueueAction"=DeviceQueue_Action."Measure_InSitu") -> (w456:T6)
        n193 = Enqueue Element(queue=w455, element=w456, error in (no error)=w453) -> (queue out=w454:refnum<queue>, error out=w444:errorcluster)  [unwired: 1 in, 1 out]
        n194 = Get Date/Time In Seconds() -> (seconds since 1Jan1904=w443:timestamp)
        n195 = Bundle By Name(cluster=w449, "QueueAction"=DataQueue_Action."Measure_InSituSpinCoating", "Time Stamp"=w443) -> (w450:T4)
        n196 = Enqueue Element(queue=w447, element=w450, error in (no error)=w444) -> (queue out=w446:refnum<queue>, error out=w445:errorcluster)  [unwired: 1 in, 1 out]
      }
      event "StartSpin_Button": Value Change {
        w465 = T6 {"QueueAction"=enum."TimeOut", "Numeric 1"=0.0, "Numeric 2"=0.0, "Boolean 1"=FALSE, "Boolean 2"=FALSE, "Spin Program"=[]}  # Device Queue
        n197 = event-data() -> ()  [unwired: 1 in, 6 out]
        n198 = Bundle By Name(cluster=w465, "QueueAction"=DeviceQueue_Action."Arduino_StartProgram") -> (w464:T6)
        n199 = Enqueue Element(queue=w463, element=w464, error in (no error)=w459) -> (queue out=w461:refnum<queue>, error out=w460:errorcluster)  [unwired: 1 in, 1 out]
      }
      event "Milliseconds": Value Change {
        w474 = T6 {"QueueAction"=enum."TimeOut", "Numeric 1"=0.0, "Numeric 2"=0.0, "Boolean 1"=FALSE, "Boolean 2"=FALSE, "Spin Program"=[]}  # Device Queue
        n200 = event-data() -> ()  [unwired: 1 in, 6 out]
        n201 = Bundle By Name(cluster=w474, "QueueAction"=DeviceQueue_Action."Arduino_SetMillis", "Numeric 1"="Milliseconds") -> (w470:T6)
        n202 = Enqueue Element(queue=w473, element=w470, error in (no error)=w471) -> (queue out=w469:refnum<queue>, error out=w468:errorcluster)  [unwired: 1 in, 1 out]
      }
      event "Speed": Value Change {
        w483 = T6 {"QueueAction"=enum."TimeOut", "Numeric 1"=0.0, "Numeric 2"=0.0, "Boolean 1"=FALSE, "Boolean 2"=FALSE, "Spin Program"=[]}  # Device Queue
        n203 = event-data() -> ()  [unwired: 1 in, 6 out]
        n204 = Bundle By Name(cluster=w483, "QueueAction"=DeviceQueue_Action."Arduino_SetSpeed", "Numeric 1"="Speed") -> (w479:T6)
        n205 = Enqueue Element(queue=w482, element=w479, error in (no error)=w480) -> (queue out=w478:refnum<queue>, error out=w477:errorcluster)  [unwired: 1 in, 1 out]
      }
      event "Debug": Value Change {
        n206 = event-data() -> ()  [unwired: 1 in, 6 out]
        n207 = Select(t=u8 0, s="Debug", f=u8 2) -> (s? t:f=w484:u8)
        n208 = property on="Milliseconds" class="DigNum (strict)"("DisabledEnum"=w484) -> ()  [unwired: 2 in, 2 out]
        n209 = property on="Speed" class="DigNum (strict)"("DisabledEnum"=w484) -> ()  [unwired: 2 in, 2 out]
      }
    }
  }
  n210 = while {
    shift-right: [w495] -> _
    shift-left: w3 -> [w499]
    shift-right: [w496] -> w5
    shift-left: w7 -> [w498]
    shift-right: [w493] -> w4
    shift-left: w2 -> [w494]
    shift-right: [w491] -> _
    shift-left: w6 -> [w492]
    stop <- w497 stop-if-true
    # "Consumer Devices"
    n211 = case shown="No Error" w499 {
      selector: w499 -> [w511 w961]
      tunnel: w498 -> [w512 w962]
      tunnel: [w508 _] -> w497
      tunnel: [w507 w962] -> w496
      tunnel: [w505 w958] -> w495
      tunnel: w494 -> [w503 w956]
      tunnel: [w504 w956] -> w493
      tunnel: w492 -> [w502 w957]
      tunnel: [w501 w957] -> w491
      frame No Error {
        n212 = Dequeue Element(queue=w512, error in (no error)=w511) -> (queue out=w510:refnum<queue>, element=w500:T6, error out=w506:errorcluster)  [unwired: 1 in, 1 out]
        n213 = Unbundle By Name(w500) -> ("QueueAction"=w509:T7)
        n214 = case shown="\"Spectrometer_GetData\"" w509 {
          tunnel: w510 -> [w516 w536 w542 w551 w600 w614 w621 w651 w658 w690 w725 w755 w778 w799 w809 w821 w833 w844 w860 w862 w869 w885 w898 w909 w945]
          tunnel: [_ w538 _ _ _ _ _ _ _ _ _ _ _ _ _ _ _ _ _ _ _ _ _ _ _] -> w508
          tunnel: [w516 w521 w542 w550 w600 w614 w622 w651 w658 w690 w724 w755 w778 w799 w809 w821 w826 w844 w860 w862 w869 w885 w898 w909 w911] -> w507
          tunnel: w506 -> [w515 w520 w543 w562 w601 w613 w636 w654 w662 w687 w731 w753 w769 w790 w806 w817 w841 w848 w859 w864 w876 w886 w897 w902 w948]
          tunnel: [w515 w519 w541 w549 w595 w612 w623 w652 w659 w673 w723 w752 w768 w789 w804 w811 w825 w847 w855 w863 w870 w884 w893 w901 w912] -> w505
          tunnel: [w513 w518 w546 w547 w597 w609 w630 w650 w657 w667 w733 w756 w761 w782 w800 w813 w839 w846 w857 w868 w880 w882 w899 w904 w910] -> w504
          tunnel: w503 -> [w513 w518 w546 w548 w597 w610 w631 w650 w657 w668 w733 w756 w764 w785 w800 w815 w839 w846 w857 w868 w880 w882 w899 w905 w910]
          tunnel: w502 -> [w514 w517 w545 w559 w599 w611 w620 w649 w661 w669 w722 w749 w760 w781 w803 w810 w838 w845 w856 w867 w879 w881 w896 w903 w950]
          tunnel: [w514 w517 w545 w553 w598 w611 w619 w647 w656 w669 w720 w750 w759 w780 w801 w810 w836 w845 w856 w867 w879 w881 w896 w903 w950] -> w501
          tunnel: w500 -> [_ _ _ _ _ _ _ _ _ w689 w728 w757 _ _ w807 _ _ _ w854 _ w877 w883 _ _ _]
          frame "TimeOut", Default {
          }
          frame "Close_Program" {
            w537 = T6 {"QueueAction"=enum."TimeOut", "Numeric 1"=0.0, "Numeric 2"=0.0, "Boolean 1"=FALSE, "Boolean 2"=FALSE, "Spin Program"=[]}  # Device Queue
            n215 = Bundle By Name(cluster=w537, "QueueAction"=DeviceQueue_Action."Spectrometer_Close") -> (w532:T6)
            n216 = Bundle By Name(cluster=w532, "QueueAction"=DeviceQueue_Action."Laser_Close") -> (w530:T6)
            n217 = Bundle By Name(cluster=w530, "QueueAction"=DeviceQueue_Action."Arduino_Close") -> (w524:T6)
            n218 = Enqueue Element(queue=w536, element=w532, error in (no error)=w520) -> (queue out=w534:refnum<queue>, error out=w529:errorcluster)  [unwired: 1 in, 1 out]
            n219 = Bundle By Name(cluster=w524, "QueueAction"=DeviceQueue_Action."Close_Program") -> (w522:T6)
            n220 = Enqueue Element(queue=w534, element=w530, error in (no error)=w529) -> (queue out=w528:refnum<queue>, error out=w527:errorcluster)  [unwired: 1 in, 1 out]
            n221 = Enqueue Element(queue=w528, element=w524, error in (no error)=w527) -> (queue out=w526:refnum<queue>, error out=w525:errorcluster)  [unwired: 1 in, 1 out]
            n222 = Enqueue Element(queue=w526, element=w522, error in (no error)=w525) -> (queue out=w521:refnum<queue>, error out=w519:errorcluster)  [unwired: 1 in, 1 out]
            n223 = First Call?() -> (First Call?: T/F=w539:bool)
            n224 = Not(x=w539) -> (.not. x?=w538:bool)
          }
          frame "Abort" {
            n225 = Unbundle By Name(w545) -> ("Port Arduino"=w544:refnum<visa-resource-name>)
            n226 = VISA Write(VISA resource name=w544, write buffer="abo", error in (no error)=w543) -> (error out=w541:errorcluster)  [unwired: 2 out]
          }
          frame "Spectrometer_Init" {
            n227 = call-dynamic "Init.vi"("error in (no error)"=w562, "Variant"=0, "Avantes in"=refnum<class "Avantes.lvclass"> refnum ("Avantes.lvclass")) -> ("error out"=w561:errorcluster, "Avantes out"=w560:refnum<class "Avantes.lvclass">)  [unwired: 7 in]
            n228 = call-dynamic "IsInit.vi"("error in (no error)"=w561, "Avantes in"=w560) -> ("error out"=w557:errorcluster, "Is Init?"=w556:bool, "Avantes out"=w558:refnum<class "Avantes.lvclass">)  [unwired: 7 in]
            n229 = property on="Spectromter" class="Bool (strict)"("Value"=w556) -> ()  [unwired: 2 in, 2 out]
            n230 = property on="Init_Spectrometer" class="Bool (strict)"("Value"=w556) -> ()  [unwired: 2 in, 2 out]
            n231 = call-dynamic "Set_ExposurePerFrame.vi"("error in (no error)"=w557, "Exposure per Frame"=1, "Avantes in"=w558) -> ("error out"=w552:errorcluster, "Avantes out"=w555:refnum<class "Avantes.lvclass">)  [unwired: 7 in]
            n232 = case shown="True" w556 {
              tunnel: w555 -> [_ w578]
              tunnel: w552 -> [w567 w576]
              tunnel: [refnum<class "Abstract_CCD.lvclass"> refnum ("Abstract_CCD.lvclass") w577] -> w554
              tunnel: w551 -> [w568 w593]
              tunnel: [w568 w582] -> w550
              tunnel: [w567 w581] -> w549
              tunnel: w548 -> [w566 w573]
              tunnel: [w566 w571] -> w547
              frame False {
              }
              frame True {
                w579 = T4 {"QueueAction"=enum."TimeOut", "Data"=[], "Data_Raw"=[], "Data_Dark"=[], "Data_Ref"=[], "Device Information"=[], "Numeric Control"=0.0, "Boolean"=FALSE, "Wavelength"=[], "Time"=[], "Time Stamp"=timestamp(0 s since 1904-01-01), "Numeric Control 2"=0.0}  # DataQueue
                w594 = T6 {"QueueAction"=enum."TimeOut", "Numeric 1"=0.0, "Numeric 2"=0.0, "Boolean 1"=FALSE, "Boolean 2"=FALSE, "Spin Program"=[]}  # Device Queue
                n233 = call-dynamic "Get_WavelengthAxis.vi"("error in (no error)"=w576, "Avantes in"=w578) -> ("error out"=w575:errorcluster, "lambda"=w570:dbl[unit][], "Avantes out"=w577:refnum<class "Avantes.lvclass">)  [unwired: 7 in]
                n234 = property on="Calculate Frames" class="Bool (strict)"() -> ("Value"=w586:bool)  [unwired: 2 in, 2 out]
                n235 = property on="Integration Time" class="DigNum (strict)"() -> ("Value"=w591:dbl[unit])  [unwired: 2 in, 2 out]
                n236 = Unbundle(w575) -> ("status"=w574:bool)  [unwired: 2 out]
                n237 = node(w591) -> (w590:dbl)
                n238 = Bundle By Name(cluster=w594, "QueueAction"=DeviceQueue_Action."Spectrometer_SetIntegrationTime", "Numeric 1"=w590, "Boolean 1"=w586) -> (w588:T6)
                n239 = property on="Frames" class="DigNum (strict)"() -> ("Value"=w585:i32)  [unwired: 2 in, 2 out]
                n240 = property on="Error_Spectromter" class="Bool (strict)"("Value"=w574) -> ()  [unwired: 2 in, 2 out]
                n241 = Enqueue Element(queue=w593, element=w588, error in (no error)=w576) -> (queue out=w589:refnum<queue>, error out=w583:errorcluster)  [unwired: 1 in, 1 out]
                n242 = Bundle By Name(cluster=w588, "QueueAction"=DeviceQueue_Action."Spectrometer_SetFrames", "Numeric 1"=w585) -> (w584:T6)
                n243 = Bundle By Name(cluster=w579, "QueueAction"=DataQueue_Action."Set_Wavelength", "Wavelength"=w570) -> (w580:T4)
                n244 = Enqueue Element(queue=w573, element=w580) -> (queue out=w571:refnum<queue>)  [unwired: 2 in, 2 out]
                n245 = Enqueue Element(queue=w589, element=w584, error in (no error)=w583) -> (queue out=w582:refnum<queue>, error out=w581:errorcluster)  [unwired: 1 in, 1 out]
              }
            }
            n246 = Bundle By Name(cluster=w559, "Abstract_CCD.lvclass"=w554) -> (w553:T3)
          }
          frame "Spectrometer_Close" {
            n247 = Unbundle By Name(w599) -> ("Abstract_CCD.lvclass"=w602:refnum<class "Abstract_CCD.lvclass">)
            n248 = flat-sequence {
              tunnel: [refnum<class "Abstract_CCD.lvclass"> refnum ("Abstract_CCD.lvclass")] -> w596
              tunnel: w595 -> [_]
              frame #0 {
              }
            }
            n249 = call-dynamic "Close.vi"("error in (no error)"=w601, "Abstract_CCD in"=w602) -> ("error out"=w595:errorcluster)  [unwired: 8 in, 1 out]
            n250 = Bundle By Name(cluster=w599, "Abstract_CCD.lvclass"=w596) -> (w598:T3)
          }
          frame "Spectrometer_Measure" {
            w616 = T4 {"QueueAction"=enum."TimeOut", "Data"=[], "Data_Raw"=[], "Data_Dark"=[], "Data_Ref"=[], "Device Information"=[], "Numeric Control"=0.0, "Boolean"=FALSE, "Wavelength"=[], "Time"=[], "Time Stamp"=timestamp(0 s since 1904-01-01), "Numeric Control 2"=0.0}  # DataQueue
            n251 = Unbundle By Name(w611) -> ("Abstract_CCD.lvclass"=w615:refnum<class "Abstract_CCD.lvclass">)
            n252 = call-dynamic "Measure.vi"("error in (no error)"=w613, "Abstract_CCD in"=w615) -> ("error out"=w612:errorcluster, "Data Raw"=w606:T9, "Data"=w607:T9, "Darkspec"=w605:T9, "Time"=w604:dbl[])  [unwired: 3 in, 2 out]
            n253 = Bundle By Name(cluster=w616, "QueueAction"=DataQueue_Action."TimeOut", "Data"=w607, "Data_Raw"=w606, "Data_Dark"=w605, "Time"=w604) -> (w617:T4)
            n254 = Enqueue Element(queue=w610, element=w617) -> (queue out=w609:refnum<queue>)  [unwired: 2 in, 2 out]
          }
          frame "Spectrometer_Preview" {
            w632 = T4 {"QueueAction"=enum."TimeOut", "Data"=[], "Data_Raw"=[], "Data_Dark"=[], "Data_Ref"=[], "Device Information"=[], "Numeric Control"=0.0, "Boolean"=FALSE, "Wavelength"=[], "Time"=[], "Time Stamp"=timestamp(0 s since 1904-01-01), "Numeric Control 2"=0.0}  # DataQueue
            n255 = Unbundle By Name(w620) -> ("Abstract_CCD.lvclass"=w637:refnum<class "Abstract_CCD.lvclass">)
            n256 = call-dynamic "Get_Frames.vi"("error in (no error)"=w636, "Abstract_CCD in"=w637) -> ("error out"=w638:errorcluster, "Numeric"=w624:i32, "Abstract_CCD out"=w639:refnum<class "Abstract_CCD.lvclass">)  [unwired: 7 in]
            n257 = call-dynamic "Set_Frames.vi"("error in (no error)"=w638, "Frames"=1, "Abstract_CCD in"=w639) -> ("error out"=w635:errorcluster, "Abstract_CCD out"=w640:refnum<class "Abstract_CCD.lvclass">)  [unwired: 7 in]
            n258 = call-dynamic "Measure.vi"("error in (no error)"=w635, "Abstract_CCD in"=w640) -> ("error out"=w626:errorcluster, "Data Raw"=w629:T9, "Abstract_CCD out"=w625:refnum<class "Abstract_CCD.lvclass">)  [unwired: 3 in, 4 out]
            n259 = property on="Preview" class="Bool (strict)"() -> ("Value"=w627:bool)  [unwired: 2 in, 2 out]
            n260 = call-dynamic "Set_Frames.vi"("error in (no error)"=w626, "Frames"=w624, "Abstract_CCD in"=w625) -> ("error out"=w623:errorcluster, "Abstract_CCD out"=w618:refnum<class "Abstract_CCD.lvclass">)  [unwired: 7 in]
            n261 = case shown="True" w627 {
              tunnel: [w641 w643] -> w622
              tunnel: w621 -> [w641 w642]
              frame False {
              }
              frame True {
                w645 = T6 {"QueueAction"=enum."TimeOut", "Numeric 1"=0.0, "Numeric 2"=0.0, "Boolean 1"=FALSE, "Boolean 2"=FALSE, "Spin Program"=[]}  # Device Queue
                n262 = Bundle By Name(cluster=w645, "QueueAction"=DeviceQueue_Action."Spectrometer_Preview") -> (w644:T6)
                n263 = Enqueue Element(queue=w642, element=w644) -> (queue out=w643:refnum<queue>)  [unwired: 2 in, 2 out]
              }
            }
            n264 = Bundle By Name(cluster=w632, "Data_Raw"=w629, "QueueAction"=DataQueue_Action."Spectrometer_Measure") -> (w633:T4)
            n265 = Enqueue Element(queue=w631, element=w633) -> (queue out=w630:refnum<queue>)  [unwired: 2 in, 2 out]
            n266 = Bundle By Name(cluster=w620, "Abstract_CCD.lvclass"=w618) -> (w619:T3)
          }
          frame "Spectrometer_StartMeasurement" {
            n267 = Unbundle By Name(w649) -> ("Abstract_CCD.lvclass"=w653:refnum<class "Abstract_CCD.lvclass">)
            n268 = call-dynamic "StartMeasure.vi"("error in (no error)"=w654, "Frames"=-1, "Abstract_CCD in"=w653) -> ("error out"=w652:errorcluster, "Abstract_CCD out"=w648:refnum<class "Abstract_CCD.lvclass">)  [unwired: 7 in]
            n269 = Bundle By Name(cluster=w649, "Abstract_CCD.lvclass"=w648) -> (w647:T3)
          }
          frame "Spectrometer_StopMeasurement" {
            n270 = Unbundle By Name(w661) -> ("Abstract_CCD.lvclass"=w663:refnum<class "Abstract_CCD.lvclass">)
            n271 = call-dynamic "StopMeasurement.vi"("error in (no error)"=w662, "Abstract_CCD in"=w663) -> ("error out"=w659:errorcluster, "Abstract_CCD out"=w660:refnum<class "Abstract_CCD.lvclass">)  [unwired: 8 in]
            n272 = Bundle By Name(cluster=w661, "Abstract_CCD.lvclass"=w660) -> (w656:T3)
          }
          frame "Spectrometer_GetData" {
            w672 = T4 {"QueueAction"=enum."TimeOut", "Data"=[], "Data_Raw"=[], "Data_Dark"=[], "Data_Ref"=[], "Device Information"=[], "Numeric Control"=0.0, "Boolean"=FALSE, "Wavelength"=[], "Time"=[], "Time Stamp"=timestamp(0 s since 1904-01-01), "Numeric Control 2"=0.0}  # DataQueue
            n273 = Unbundle By Name(w669) -> ("Abstract_CCD.lvclass"=w688:refnum<class "Abstract_CCD.lvclass">)
            n274 = Unbundle By Name(w689) -> ("Numeric 1"=w684:dbl)
            n275 = Initialize Array(nan ("element"), w684) -> (w683:dbl[])
            n276 = for {
              N: w684 -> [w697]
              tunnel: w688 -> [w707]
              shift-right: [w698] -> w673
              shift-left: w687 -> [w708]
              shift-right: [w702] -> w677
              shift-left: dbl[][][] [] -> [w701]
              shift-right: [w693] -> w664
              shift-left: w683 -> [w696]
              i -> [w695]
              w692 = 0 ("index (page)")
              n277 = call-dynamic "Measure_GetData.vi"("error in (no error)"=w708, "Abstract_CCD in"=w707) -> ("error out"=w698:errorcluster, "Data_Raw"=w706:T9, "Time"=w694:dbl[])  [unwired: 6 in, 1 out]
              n278 = Index Array(array=w706, index=0) -> (element=w704:T10)
              n279 = Unbundle(w704) -> ("Image"=w700:dbl[][][])  [unwired: 1 out]
              n280 = case shown="0" w695 {
                tunnel: w700 -> [w718 _]
                tunnel: [w710 w719] -> w703
                tunnel: w701 -> [_ w719]
                tunnel: w697 -> [w709 _]
                frame 0 {
                  n281 = Array Size(array=w718) -> (size(s)=w717:i32[])
                  n282 = Index Array(array=w717, index #1=0 ("index"), index #2=1 ("index"), index #3=2 ("index")) -> (element #2=w713:i32, element #3=w712:i32)  [unwired: 1 out]
                  n283 = Initialize Array(nan ("element"), w709, w713, w712) -> (w710:dbl[][][])
                }
                frame Default {
                }
              }
              n284 = Index Array(array=w700, index (dim 0)=w692, index (dim 1)=w692) -> (element=w699:dbl[])  [unwired: 1 in]
              n285 = Replace Array Subset(array=w696, new element=w694, index=w695) -> (w693:dbl[])
              n286 = Replace Array Subset(array=w703, new element=w699, index (dim 0)=w695, index (dim 1)=0 ("disabled index (row)")) -> (w702:dbl[][][])  [unwired: 1 in]
            }
            n287 = Array Size(array=w677) -> (size(s)=w681:i32[])
            n288 = Index Array(array=w681, index #1=0 ("index"), index #2=1 ("index"), index #3=2 ("index")) -> (element #1=w676:i32, element #2=w675:i32, element #3=w674:i32)
            n289 = Bundle By Name(cluster=T10 {"Image"=[], "Frame Size"={"F"=0, "Y"=0, "X"=0}} ("Cluster"), "Image"=w677, "Frame Size.F"=w676, "Frame Size.Y"=w675, "Frame Size.X"=w674) -> (w666:T10)
            n290 = Build Array(w666) -> (w665:T9)
            n291 = Bundle By Name(cluster=w672, "QueueAction"=DataQueue_Action."Spectrometer_Measure", "Data_Raw"=w665, "Time"=w664) -> (w671:T4)
            n292 = Enqueue Element(queue=w668, element=w671) -> (queue out=w667:refnum<queue>)  [unwired: 2 in, 2 out]
          }
          frame "Spectrometer_SetIntegrationTime" {
            n293 = Unbundle By Name(w728) -> ("Numeric 1"=w730:dbl)
            n294 = Unbundle By Name(w722) -> ("Abstract_CCD.lvclass"=w732:refnum<class "Abstract_CCD.lvclass">)
            n295 = Unbundle By Name(w728) -> ("Boolean 1"=w727:bool)
            n296 = node(w730) -> (w729:dbl[unit])
            n297 = call-dynamic "Set_ExposureTime.vi"("error in (no error)"=w731, "Exposure Time"=w729, "Abstract_CCD in"=w732) -> ("error out"=w735:errorcluster, "Abstract_CCD out"=w734:refnum<class "Abstract_CCD.lvclass">)  [unwired: 7 in]
            n298 = call-dynamic "Get_FrameRate.vi"("error in (no error)"=w735, "Abstract_CCD in"=w734) -> ("error out"=w723:errorcluster, "Frame Rate"=w726:dbl[unit], "Abstract_CCD out"=w721:refnum<class "Abstract_CCD.lvclass">)  [unwired: 7 in]
            "Frame Rate" <- w726
            n299 = Bundle By Name(cluster=w722, "Abstract_CCD.lvclass"=w721) -> (w720:T3)
            n300 = case shown="True" w727 {
              tunnel: w726 -> [_ w744]
              tunnel: w725 -> [w736 w738]
              tunnel: [w736 w737] -> w724
              frame False {
              }
              frame True {
                w742 = T6 {"QueueAction"=enum."TimeOut", "Numeric 1"=0.0, "Numeric 2"=0.0, "Boolean 1"=FALSE, "Boolean 2"=FALSE, "Spin Program"=[]}  # Device Queue
                n301 = property on="Program Spin Coater\nSpeed (rpm)          Time (s)" class="Arr (strict)"() -> ("Value"=w747:dbl[][])  [unwired: 2 in, 2 out]
                n302 = property on="Seconds to Spin Start" class="DigNum (strict)"() -> ("Value"=w746:dbl[unit])  [unwired: 2 in, 2 out]
                n303 = property on="Seconds after Spin Stop" class="DigNum (strict)"() -> ("Value"=w745:dbl[unit])  [unwired: 2 in, 2 out]
                n304 = call "CalculateFrames.vi"("Program Spin Coater\nSpeed (rpm)          Time (s)"=w747, "Seconds End"=w745, "Seconds Start"=w746, "Frame Rate"=w744) -> ("Time"=w743:dbl, "Frames"=w739:i32)  [unwired: 6 in]
                n305 = property on="Overall Time" class="DigNum (strict)"("Value"=w743) -> ()  [unwired: 2 in, 2 out]
                n306 = Bundle By Name(cluster=w742, "QueueAction"=DeviceQueue_Action."Spectrometer_SetFrames", "Numeric 1"=w739) -> (w741:T6)
                n307 = Enqueue Element(queue=w738, element=w741) -> (queue out=w737:refnum<queue>)  [unwired: 2 in, 2 out]
              }
            }
          }
          frame "Spectrometer_SetFrames" {
            n308 = Unbundle By Name(w749) -> ("Abstract_CCD.lvclass"=w754:refnum<class "Abstract_CCD.lvclass">)
            n309 = Unbundle By Name(w757) -> ("Numeric 1"=w751:dbl)
            n310 = property on="Frames" class="DigNum (strict)"("Value"=w751) -> ()  [unwired: 2 in, 2 out]
            n311 = call-dynamic "Set_Frames.vi"("error in (no error)"=w753, "Frames"=w751, "Abstract_CCD in"=w754) -> ("error out"=w752:errorcluster, "Abstract_CCD out"=w748:refnum<class "Abstract_CCD.lvclass">)  [unwired: 7 in]
            n312 = Bundle By Name(cluster=w749, "Abstract_CCD.lvclass"=w748) -> (w750:T3)
          }
          frame "Spectrometer_SetDarkspec" {
            w765 = T4 {"QueueAction"=enum."TimeOut", "Data"=[], "Data_Raw"=[], "Data_Dark"=[], "Data_Ref"=[], "Device Information"=[], "Numeric Control"=0.0, "Boolean"=FALSE, "Wavelength"=[], "Time"=[], "Time Stamp"=timestamp(0 s since 1904-01-01), "Numeric Control 2"=0.0}  # DataQueue
            n313 = Unbundle By Name(w760) -> ("Abstract_CCD.lvclass"=w777:refnum<class "Abstract_CCD.lvclass">)
            n314 = property on="Frames for Dark/Ref" class="DigNum (strict)"() -> ("Value"=w767:dbl)  [unwired: 2 in, 2 out]
            n315 = call-dynamic "Get_Frames.vi"("error in (no error)"=w769, "Abstract_CCD in"=w777) -> ("error out"=w774:errorcluster, "Numeric"=w775:i32, "Abstract_CCD out"=w776:refnum<class "Abstract_CCD.lvclass">)  [unwired: 7 in]
            n316 = call-dynamic "Set_Frames.vi"("error in (no error)"=w774, "Frames"=w767, "Abstract_CCD in"=w776) -> ("error out"=w773:errorcluster, "Abstract_CCD out"=w770:refnum<class "Abstract_CCD.lvclass">)  [unwired: 7 in]
            n317 = call-dynamic "Measure.vi"("error in (no error)"=w773, "Abstract_CCD in"=w770) -> ("error out"=w772:errorcluster, "Data Raw"=w762:T9, "Abstract_CCD out"=w771:refnum<class "Abstract_CCD.lvclass">)  [unwired: 3 in, 4 out]
            n318 = call-dynamic "Set_Frames.vi"("error in (no error)"=w772, "Frames"=w775, "Abstract_CCD in"=w771) -> ("error out"=w768:errorcluster, "Abstract_CCD out"=w758:refnum<class "Abstract_CCD.lvclass">)  [unwired: 7 in]
            n319 = Bundle By Name(cluster=w765, "QueueAction"=DataQueue_Action."Set_Dark", "Data_Dark"=w762) -> (w766:T4)
            n320 = Enqueue Element(queue=w764, element=w766) -> (queue out=w761:refnum<queue>)  [unwired: 2 in, 2 out]
            n321 = Bundle By Name(cluster=w760, "Abstract_CCD.lvclass"=w758) -> (w759:T3)
          }
          frame "Spectrometer_SetReference" {
            w786 = T4 {"QueueAction"=enum."TimeOut", "Data"=[], "Data_Raw"=[], "Data_Dark"=[], "Data_Ref"=[], "Device Information"=[], "Numeric Control"=0.0, "Boolean"=FALSE, "Wavelength"=[], "Time"=[], "Time Stamp"=timestamp(0 s since 1904-01-01), "Numeric Control 2"=0.0}  # DataQueue
            n322 = Unbundle By Name(w781) -> ("Abstract_CCD.lvclass"=w798:refnum<class "Abstract_CCD.lvclass">)
            n323 = property on="Frames for Dark/Ref" class="DigNum (strict)"() -> ("Value"=w788:dbl)  [unwired: 2 in, 2 out]
            n324 = call-dynamic "Get_Frames.vi"("error in (no error)"=w790, "Abstract_CCD in"=w798) -> ("error out"=w795:errorcluster, "Numeric"=w796:i32, "Abstract_CCD out"=w797:refnum<class "Abstract_CCD.lvclass">)  [unwired: 7 in]
            n325 = call-dynamic "Set_Frames.vi"("error in (no error)"=w795, "Frames"=w788, "Abstract_CCD in"=w797) -> ("error out"=w794:errorcluster, "Abstract_CCD out"=w791:refnum<class "Abstract_CCD.lvclass">)  [unwired: 7 in]
            n326 = call-dynamic "Measure.vi"("error in (no error)"=w794, "Abstract_CCD in"=w791) -> ("error out"=w793:errorcluster, "Data Raw"=w783:T9, "Abstract_CCD out"=w792:refnum<class "Abstract_CCD.lvclass">)  [unwired: 3 in, 4 out]
            n327 = call-dynamic "Set_Frames.vi"("error in (no error)"=w793, "Frames"=w796, "Abstract_CCD in"=w792) -> ("error out"=w789:errorcluster, "Abstract_CCD out"=w779:refnum<class "Abstract_CCD.lvclass">)  [unwired: 7 in]
            n328 = Bundle By Name(cluster=w786, "QueueAction"=DataQueue_Action."Set_Ref", "Data_Ref"=w783) -> (w787:T4)
            n329 = Enqueue Element(queue=w785, element=w787) -> (queue out=w782:refnum<queue>)  [unwired: 2 in, 2 out]
            n330 = Bundle By Name(cluster=w781, "Abstract_CCD.lvclass"=w779) -> (w780:T3)
          }
          frame "Spectrometer_SetTriggerMode" {
            n331 = Unbundle By Name(w803) -> ("Abstract_CCD.lvclass"=w808:refnum<class "Abstract_CCD.lvclass">)
            n332 = Unbundle By Name(w807) -> ("Numeric 1"=w805:dbl)
            n333 = call-dynamic "Set_TriggerMode.vi"("error in (no error)"=w806, "Trigger Mode"=w805, "Abstract_CCD in"=w808) -> ("error out"=w804:errorcluster, "Abstract_CCD out"=w802:refnum<class "Abstract_CCD.lvclass">)  [unwired: 7 in]
            n334 = Bundle By Name(cluster=w803, "Abstract_CCD.lvclass"=w802) -> (w801:T3)
          }
          frame "Spectrometer_DeviceInformation" {
            w816 = T4 {"QueueAction"=enum."TimeOut", "Data"=[], "Data_Raw"=[], "Data_Dark"=[], "Data_Ref"=[], "Device Information"=[], "Numeric Control"=0.0, "Boolean"=FALSE, "Wavelength"=[], "Time"=[], "Time Stamp"=timestamp(0 s since 1904-01-01), "Numeric Control 2"=0.0}  # DataQueue
            n335 = Unbundle By Name(w810) -> ("Abstract_CCD.lvclass"=w818:refnum<class "Abstract_CCD.lvclass">)
            n336 = call-dynamic "Get_DeviceInformation.vi"("error in (no error)"=w817, "Abstract_CCD in"=w818) -> ("error out"=w812:errorcluster, "Array"=w819:string[])  [unwired: 7 in, 1 out]
            n337 = Bundle By Name(cluster=w816, "QueueAction"=DataQueue_Action."Transfer_Settings", "Device Information"=w819) -> (w814:T4)
            n338 = Enqueue Element(queue=w815, element=w814, error in (no error)=w812) -> (queue out=w813:refnum<queue>, error out=w811:errorcluster)  [unwired: 1 in, 1 out]
          }
          frame "Arduino_Init" {
            w835 = T6 {"QueueAction"=enum."TimeOut", "Numeric 1"=0.0, "Numeric 2"=0.0, "Boolean 1"=FALSE, "Boolean 2"=FALSE, "Spin Program"=[]}  # Device Queue
            n339 = call-poly "VISA Configure Serial Port"("VISA resource name"="Port Arduino", "baud rate (9600)"=u32 115200, "error in (no error)"=w841) -> ("VISA resource name out"=w837:refnum<visa-resource-name>, "error out"=w824:errorcluster)  [unwired: 11 in]
            n340 = Unbundle(w824) -> ("status"=w823:bool)  [unwired: 2 out]
            n341 = Not(x=w823) -> (.not. x?=w822:bool)
            n342 = property on="Arduino" class="Bool (strict)"("Value"=w822) -> ()  [unwired: 2 in, 2 out]
            n343 = property on="Program Spin Coater\nSpeed (rpm)          Time (s)" class="Arr (strict)"() -> ("Value"=w830:dbl[][])  [unwired: 2 in, 2 out]
            n344 = Bundle By Name(cluster=w835, "QueueAction"=DeviceQueue_Action."Arduino_LoadProgram", "Spin Program"=dbl[][] []) -> (w831:T6)
            n345 = Enqueue Element(queue=w833, element=w831, error in (no error)=w824) -> (queue out=w829:refnum<queue>, error out=w828:errorcluster)  [unwired: 1 in, 1 out]
            n346 = Bundle By Name(cluster=w831, "Spin Program"=w830) -> (w827:T6)
            n347 = Bundle By Name(cluster=w838, "Port Arduino"=w837) -> (w836:T3)
            n348 = Enqueue Element(queue=w829, element=w827, error in (no error)=w828) -> (queue out=w826:refnum<queue>, error out=w825:errorcluster)  [unwired: 1 in, 1 out]
          }
          frame "Arduino_Close" {
            n349 = Unbundle By Name(w845) -> ("Port Arduino"=w849:refnum<visa-resource-name>)
            n350 = property on="Arduino" class="Bool (strict)"("Value"=FALSE ("Arduino")) -> ()  [unwired: 2 in, 2 out]
            n351 = VISA Close(VISA resource name=w849, error in (no error)=w848) -> (error out=w847:errorcluster)
          }
          frame "Arduino_LoadProgram" {
            n352 = Unbundle By Name(w854) -> ("Spin Program"=w853:dbl[][], "Numeric 1"=w851:dbl)
            n353 = Unbundle By Name(w856) -> ("Port Arduino"=w858:refnum<visa-resource-name>)
            n354 = node(w851) -> (w850:dbl[unit])
            n355 = call "SpinCoaterArray2String.vi"("Seconds to Spin Start"=w850, "Program Spin Coater\nSpeed (rpm)          Time (s)"=w853) -> ("remote control String"=w852:string)  [unwired: 3 in]
            n356 = VISA Write(VISA resource name=w858, write buffer=w852, error in (no error)=w859) -> (error out=w855:errorcluster)  [unwired: 2 out]
          }
          frame "Arduino_StartProgram" {
            n357 = Unbundle By Name(w867) -> ("Port Arduino"=w866:refnum<visa-resource-name>)
            n358 = VISA Write(VISA resource name=w866, write buffer="run", error in (no error)=w864) -> (error out=w863:errorcluster)  [unwired: 2 out]
            n359 = property on="Action" class="Str"("Value"="Measuring" ("Action")) -> ()  [unwired: 2 in, 2 out]
          }
          frame "Arduino_SetSpeed" {
            n360 = Unbundle By Name(w877) -> ("Numeric 1"=w875:dbl)
            n361 = Unbundle By Name(w879) -> ("Port Arduino"=w878:refnum<visa-resource-name>)
            n362 = To Unsigned Long Integer(number=w875) -> (unsigned 32bit integer=w874:u32)
            n363 = Number To Decimal String(number=w874) -> (decimal integer string=w873:string)  [unwired: 1 in]
            n364 = Concatenate Strings("!spe" ("string"), w873) -> (w871:string)
            n365 = VISA Write(VISA resource name=w878, write buffer=w871, error in (no error)=w876) -> (error out=w870:errorcluster)  [unwired: 2 out]
          }
          frame "Arduino_SetMillis" {
            n366 = Unbundle By Name(w883) -> ("Numeric 1"=w891:dbl)
            n367 = Unbundle By Name(w881) -> ("Port Arduino"=w892:refnum<visa-resource-name>)
            n368 = To Unsigned Long Integer(number=w891) -> (unsigned 32bit integer=w890:u32)
            n369 = Number To Decimal String(number=w890) -> (decimal integer string=w889:string)  [unwired: 1 in]
            n370 = Concatenate Strings("!mil" ("string"), w889) -> (w887:string)
            n371 = VISA Write(VISA resource name=w892, write buffer=w887, error in (no error)=w886) -> (error out=w884:errorcluster)  [unwired: 2 out]
          }
          frame "Arduino_StopSpin" {
            n372 = Unbundle By Name(w896) -> ("Port Arduino"=w895:refnum<visa-resource-name>)
            n373 = VISA Write(VISA resource name=w895, write buffer="abo", error in (no error)=w897) -> (error out=w893:errorcluster)  [unwired: 2 out]
          }
          frame "Measure_Stop" {
            w907 = T4 {"QueueAction"=enum."TimeOut", "Data"=[], "Data_Raw"=[], "Data_Dark"=[], "Data_Ref"=[], "Device Information"=[], "Numeric Control"=0.0, "Boolean"=FALSE, "Wavelength"=[], "Time"=[], "Time Stamp"=timestamp(0 s since 1904-01-01), "Numeric Control 2"=0.0}  # DataQueue
            n374 = Bundle By Name(cluster=w907, "QueueAction"=DataQueue_Action."Stop_Measurement") -> (w908:T4)
            n375 = Enqueue Element(queue=w905, element=w908, error in (no error)=w902) -> (queue out=w904:refnum<queue>, error out=w901:errorcluster)  [unwired: 1 in, 1 out]
            n376 = property on="StartMeasurement_Button" class="Bool (strict)"("Value"=FALSE ("StartMeasurement_Button")) -> ()  [unwired: 2 in, 2 out]
          }
          frame "Measure_InSitu" {
            w922 = 1000 ("y")
            w938 = T6 {"QueueAction"=enum."TimeOut", "Numeric 1"=0.0, "Numeric 2"=0.0, "Boolean 1"=FALSE, "Boolean 2"=FALSE, "Spin Program"=[]}  # Device Queue
            w946 = T6 {"QueueAction"=enum."TimeOut", "Numeric 1"=0.0, "Numeric 2"=0.0, "Boolean 1"=FALSE, "Boolean 2"=FALSE, "Spin Program"=[]}  # Device Queue
            n377 = Unbundle By Name(w950) -> ("Abstract_CCD.lvclass"=w949:refnum<class "Abstract_CCD.lvclass">)
            n378 = call-dynamic "Get_Frames.vi"("error in (no error)"=w948, "Abstract_CCD in"=w949) -> ("error out"=w943:errorcluster, "Numeric"=w933:i32)  [unwired: 7 in, 1 out]
            n379 = Bundle By Name(cluster=w946, "QueueAction"=DeviceQueue_Action."Spectrometer_SetTriggerMode", "Numeric 1"=1.0) -> (w944:T6)
            n380 = Bundle By Name(cluster=w938, "QueueAction"=DeviceQueue_Action."Spectrometer_DeviceInformation") -> (w935:T6)
            n381 = Bundle By Name(cluster=w935, "QueueAction"=DeviceQueue_Action."Spectrometer_StartMeasurement") -> (w930:T6)
            n382 = Enqueue Element(queue=w945, element=w944, error in (no error)=w943) -> (queue out=w940:refnum<queue>, error out=w941:errorcluster)  [unwired: 1 in, 1 out]
            n383 = Bundle By Name(cluster=w930, "QueueAction"=DeviceQueue_Action."Arduino_StartProgram") -> (w925:T6)
            n384 = Enqueue Element(queue=w940, element=w935, error in (no error)=w941) -> (queue out=w937:refnum<queue>, error out=w936:errorcluster)  [unwired: 1 in, 1 out]
            n385 = Bundle By Name(cluster=w925, "QueueAction"=DeviceQueue_Action."Spectrometer_GetData", "Numeric 1"=w922) -> (w919:T6)
            n386 = Divide(x=w933, y=w922) -> (x/y=w932:dbl)
            n387 = Round Toward +Infinity(x=w932) -> (ceil(x): smallest int >= x=w931:dbl)
            n388 = Enqueue Element(queue=w937, element=w930, error in (no error)=w936) -> (queue out=w929:refnum<queue>, error out=w928:errorcluster)  [unwired: 1 in, 1 out]
            n389 = Enqueue Element(queue=w929, element=w925, error in (no error)=w928) -> (queue out=w926:refnum<queue>, error out=w923:errorcluster)  [unwired: 1 in, 1 out]
            n390 = for {
              N: w931 -> [_]
              shift-right: [w951] -> w921
              shift-left: w926 -> [w955]
              tunnel: w919 -> [w952]
              shift-right: [w953] -> w920
              shift-left: w923 -> [w954]
              n391 = Enqueue Element(queue=w955, element=w952, error in (no error)=w954) -> (queue out=w951:refnum<queue>, error out=w953:errorcluster)  [unwired: 1 in, 1 out]
            }
            n392 = Bundle By Name(cluster=w919, "QueueAction"=DeviceQueue_Action."Spectrometer_StopMeasurement") -> (w915:T6)
            n393 = Bundle By Name(cluster=w915, "QueueAction"=DeviceQueue_Action."Measure_Stop") -> (w913:T6)
            n394 = Enqueue Element(queue=w921, element=w915, error in (no error)=w920) -> (queue out=w916:refnum<queue>, error out=w917:errorcluster)  [unwired: 1 in, 1 out]
            n395 = Enqueue Element(queue=w916, element=w913, error in (no error)=w917) -> (queue out=w911:refnum<queue>, error out=w912:errorcluster)  [unwired: 1 in, 1 out]
          }
        }
      }
      frame Error {
        w960 = T12 4 items=["no dialog", "OK message", "continue or stop message", "OK message + warnings", "continue/stop + warnings"] ("type of dialog (OK msg:1)")
        n396 = call <vilib>:"General Error Handler.vi"("type of dialog (OK msg:1)"=w960, "error in (no error)"=w961) -> ("error out"=w959:errorcluster)  [unwired: 9 in, 4 out]
        n397 = call <vilib>:"Clear Errors.vi"("error in (no error)"=w959) -> ("error out"=w958:errorcluster)  [unwired: 5 in, 1 out]
      }
    }
  }
  n398 = Release Queue(queue=w4) -> ()  [unwired: 2 in, 3 out]
  n399 = Release Queue(queue=w5) -> ()  [unwired: 2 in, 3 out]
